vi "日志信息出发送队列 (子VI).vi"() -> (0 "错误输出":errorcluster)   [LabVIEW 2016, in "数据传输系统-05.lvlib"]
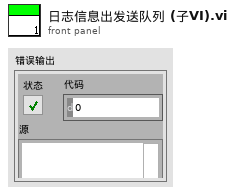
[diagram p1: front panel]
types:
  T1 = enum16{"空白测试", "跨度核查", "标样核查", "加标回收", "平行样", "集成干预"}
  T2 = cluster{"氨氮零点核查索引起始时间":string, "总磷零点核查索引起始时间":string, "总氮零点核查索引起始时间":string, "CODMn零点核查索引起始时间":string, "CODCr零点核查索引起始时间":string, "亚硝酸盐零点核查索引起始时间":string, "硫化物零点核查索引起始时间":string, "ORP零点核查索引起始时间":string, "氟化物零点核查索引起始时间":string}
  T3 = cluster{"数组[0]":string, "数组[1]":string, "数组[2]":string, "数组[3]":string, "数组[4]":string, "数组[5]":string, "数组[6]":string, "数组[7]":string, "数组[8]":string}
  T4 = cluster{"PH":string[][], "CODCr":string[][], "氨氮":string[][], "CODMn":string[][], "总氮":string[][], "总磷":string[][], "电导率":string[][], "水温":string[][], "DO":string[][], "浊度":string[][], "叶绿素":string[][], "藻密度":string[][], "铜":string[][], "盐度":string[][], "水位":string[][], "流速":string[][], "瞬时流量":string[][], "累积流量":string[][], "亚硝酸盐":string[][], "硫化物":string[][], "ORP":string[][], "铅":string[][], "镉":string[][], "锌":string[][], "镍":string[][], "锰":string[][], "汞":string[][], "气温":string[][], "气压":string[][], "风速":string[][], "风向":string[][], "盐度 2":string[][], "磷酸盐":string[][], "硝氮":string[][], "氟化物":string[][]}
  T5 = cluster{"氨氮跨度核查索引起始时间":string, "总磷跨度核查索引起始时间":string, "总氮跨度核查索引起始时间":string, "CODMn跨度核查索引起始时间":string, "CODCr跨度核查索引起始时间":string, "亚硝酸盐跨度核查索引起始时间":string, "硫化物跨度核查索引起始时间":string, "ORP跨度核查索引起始时间":string, "氟化物跨度核查索引起始时间":string}
  T6 = cluster{"氨氮标样核查索引起始时间":string, "总磷标样核查索引起始时间":string, "总氮标样核查索引起始时间":string, "CODMn标样核查索引起始时间":string, "CODCr标样核查索引起始时间":string, "DO标样核查索引起始时间":string, "PH标样核查索引起始时间":string, "比电导率标样核查索引起始时间":string, "水温标样核查索引起始时间":string, "浊度标样核查索引起始时间":string, "叶绿素a标样核查索引起始时间":string, "藻密度标样核查索引起始时间":string, "亚硝酸盐标样核查索引起始时间":string, "硫化物标样核查索引起始时间":string, "ORP标样核查索引起始时间":string, "氟化物标样核查索引起始时间":string}
  T7 = cluster{"数组[0]":string, "数组[1]":string, "数组[2]":string, "数组[3]":string, "数组[4]":string, "数组[5]":string, "数组[6]":string, "数组[7]":string, "数组[8]":string, "数组[9]":string, "数组[10]":string, "数组[11]":string, "数组[12]":string, "数组[13]":string, "数组[14]":string, "数组[15]":string}
  T8 = cluster{"氨氮加标回收索引起始时间":string, "总磷加标回收索引起始时间":string, "总氮加标回收索引起始时间":string, "CODMn加标回收索引起始时间":string, "CODCr加标回收索引起始时间":string, "氟化物加标回收索引起始时间":string}
  T9 = cluster{"[0]":string, "[1]":string, "[2]":string, "[3]":string, "[4]":string, "[5]":string}
  T10 = cluster{"氨氮平行样索引起始时间":string, "总磷平行样索引起始时间":string, "总氮平行样索引起始时间":string, "CODMn平行样索引起始时间":string, "CODCr平行样索引起始时间":string, "氟化物平行样索引起始时间":string}
  T11 = cluster{"氨氮集成干预索引起始时间":string, "总磷集成干预索引起始时间":string, "总氮集成干预索引起始时间":string, "CODMn集成干预索引起始时间":string, "CODCr集成干预索引起始时间":string, "DO集成干预索引起始时间":string, "PH集成干预索引起始时间":string, "比电导率集成干预索引起始时间":string, "水温集成干预索引起始时间":string, "浊度集成干预索引起始时间":string, "叶绿素a集成干预索引起始时间":string, "藻密度集成干预索引起始时间":string, "亚硝酸盐集成干预索引起始时间":string, "硫化物集成干预索引起始时间":string, "ORP集成干预索引起始时间":string, "氟化物集成干预索引起始时间":string}
  T12 = cluster{"[0]":string, "[1]":string, "[2]":string, "[3]":string, "[4]":string, "[5]":string, "[6]":string, "[7]":string, "[8]":string, "[9]":string, "[10]":string, "[11]":string, "[12]":string, "[13]":string, "[14]":string, "[15]":string}
  T13 = cluster{"氨氮仪器日志索引起始时间":string, "总磷仪器日志索引起始时间":string, "总氮仪器日志索引起始时间":string, "CODMn仪器日志索引起始时间":string, "CODCr仪器日志索引起始时间":string, "系统仪器日志索引起始时间":string, "氟化物仪器日志索引起始时间":string}
  T14 = cluster{"[0]":string, "[1]":string, "[2]":string, "[3]":string, "[4]":string, "[5]":string, "[6]":string}
  T15 = cluster{"氨氮报警信息索引起始时间":string, "总磷报警信息索引起始时间":string, "总氮报警信息索引起始时间":string, "CODMn报警信息索引起始时间":string, "CODCr报警信息索引起始时间":string, "DO报警信息索引起始时间":string, "PH报警信息索引起始时间":string, "比电导率报警信息索引起始时间":string, "水温报警信息索引起始时间":string, "浊度报警信息索引起始时间":string, "叶绿素报警信息索引起始时间":string, "系统报警信息索引起始时间":string, "氟化物报警信息索引起始时间":string}
  T16 = cluster{"[0]":string, "[1]":string, "[2]":string, "[3]":string, "[4]":string, "[5]":string, "[6]":string, "[7]":string, "[8]":string, "[9]":string, "[10]":string, "[11]":string, "[12]":string}
  T17 = cluster{"氨氮仪器参数索引起始时间":string, "总磷仪器参数索引起始时间":string, "总氮仪器参数索引起始时间":string, "CODMn仪器参数索引起始时间":string, "CODCr仪器参数索引起始时间":string, "DO仪器参数索引起始时间":string, "PH仪器参数索引起始时间":string, "比电导率仪器参数索引起始时间":string, "水温仪器参数索引起始时间":string, "浊度仪器参数索引起始时间":string, "叶绿素a仪器参数索引起始时间":string, "藻密度仪器参数索引起始时间":string, "ORP仪器参数索引起始时间":string, "氟化物仪器参数索引起始时间":string}
  T18 = cluster{"[0]":string, "[1]":string, "[2]":string, "[3]":string, "[4]":string, "[5]":string, "[6]":string, "[7]":string, "[8]":string, "[9]":string, "[10]":string, "[11]":string, "[12]":string, "[13]":string}
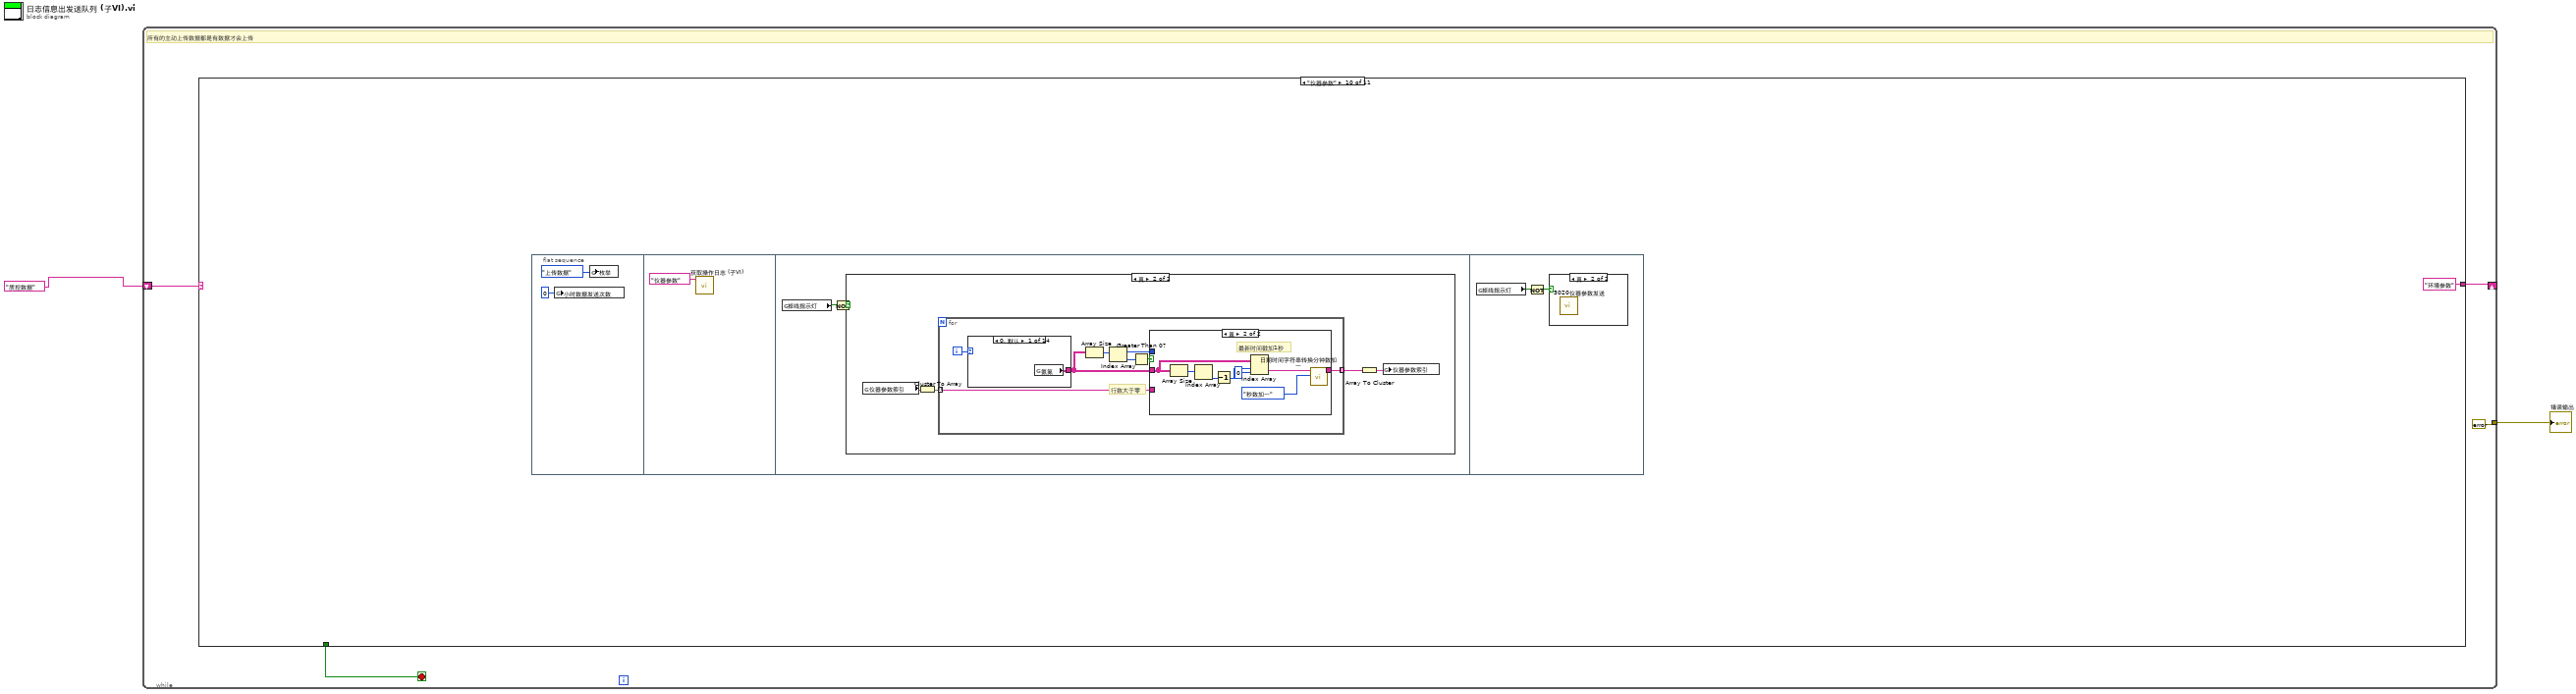
[diagram p0: block diagram]
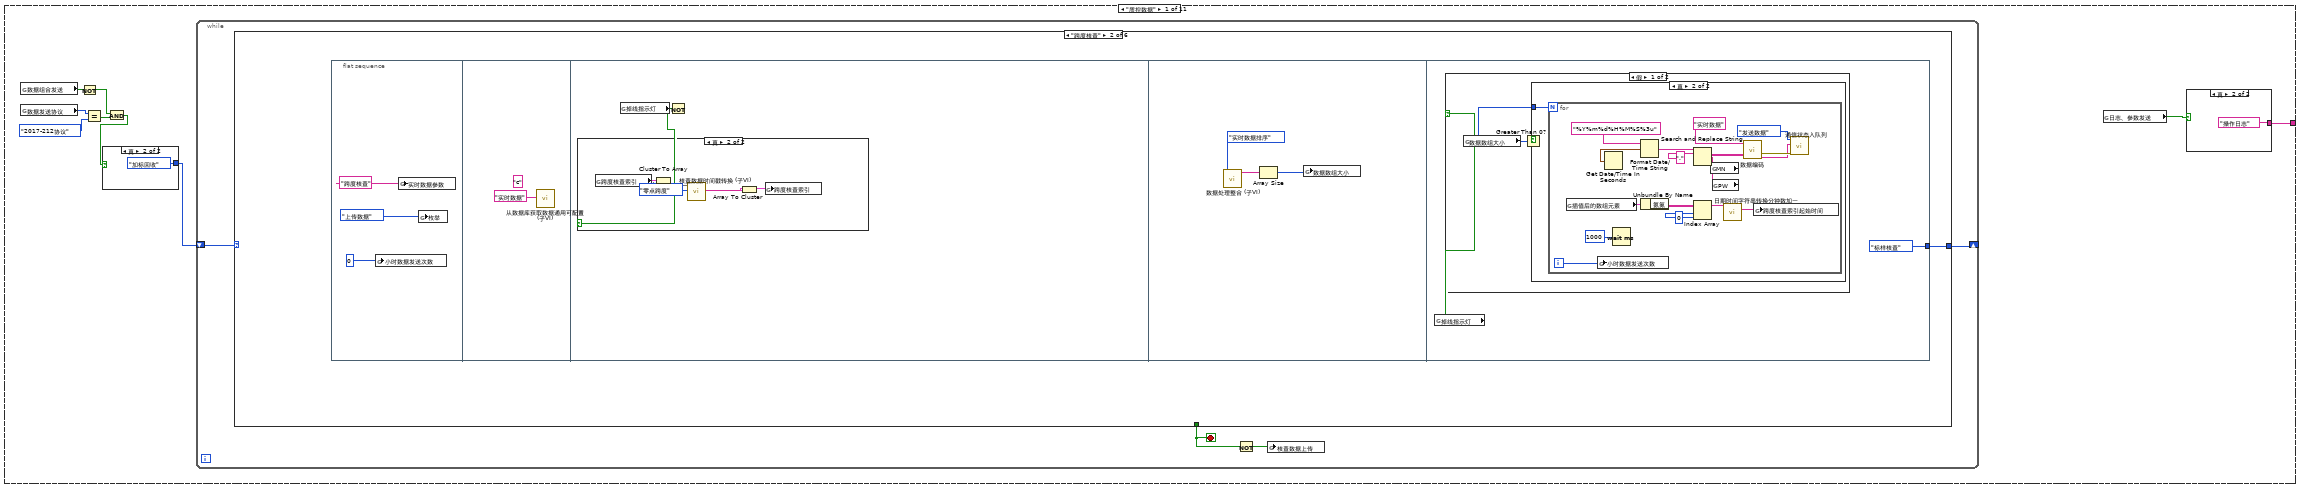
[diagram p2: hidden frame]
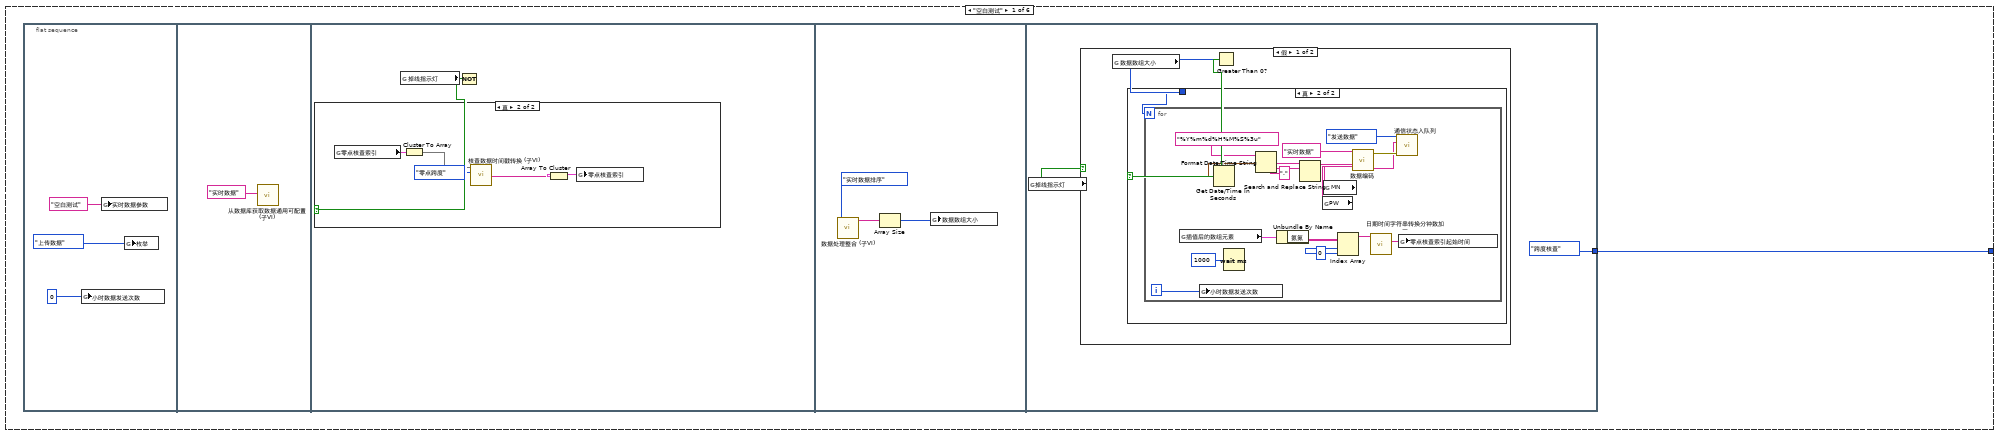
[diagram p3: hidden frame]
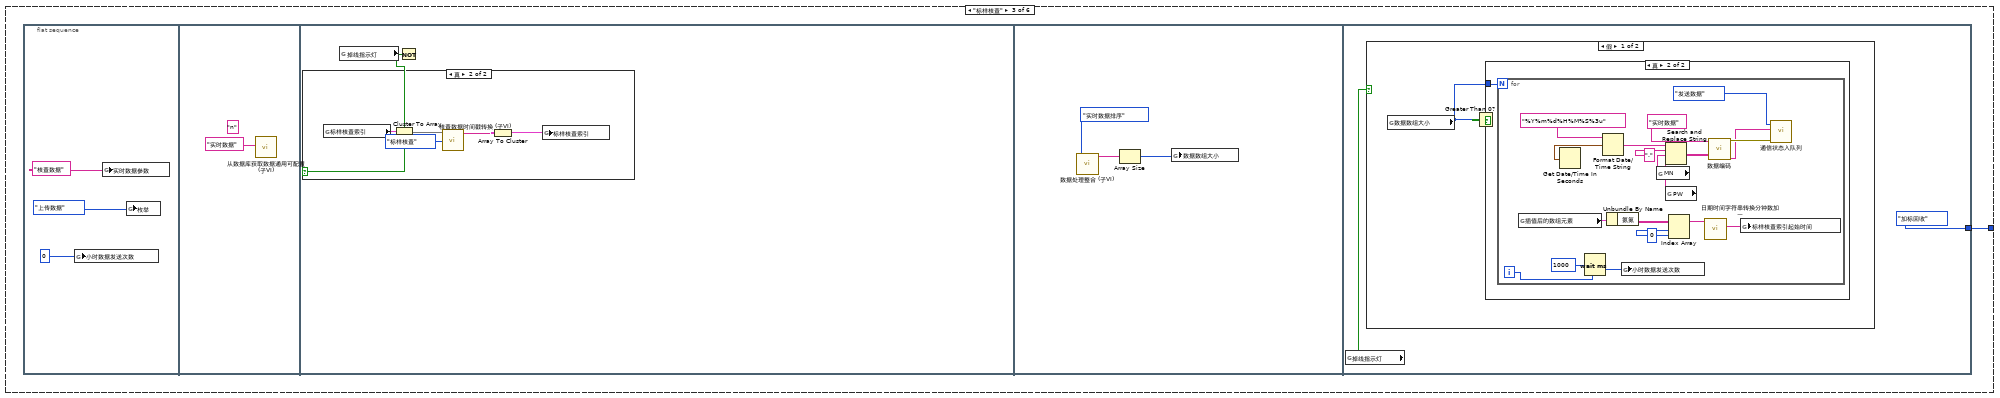
[diagram p10: hidden frame]
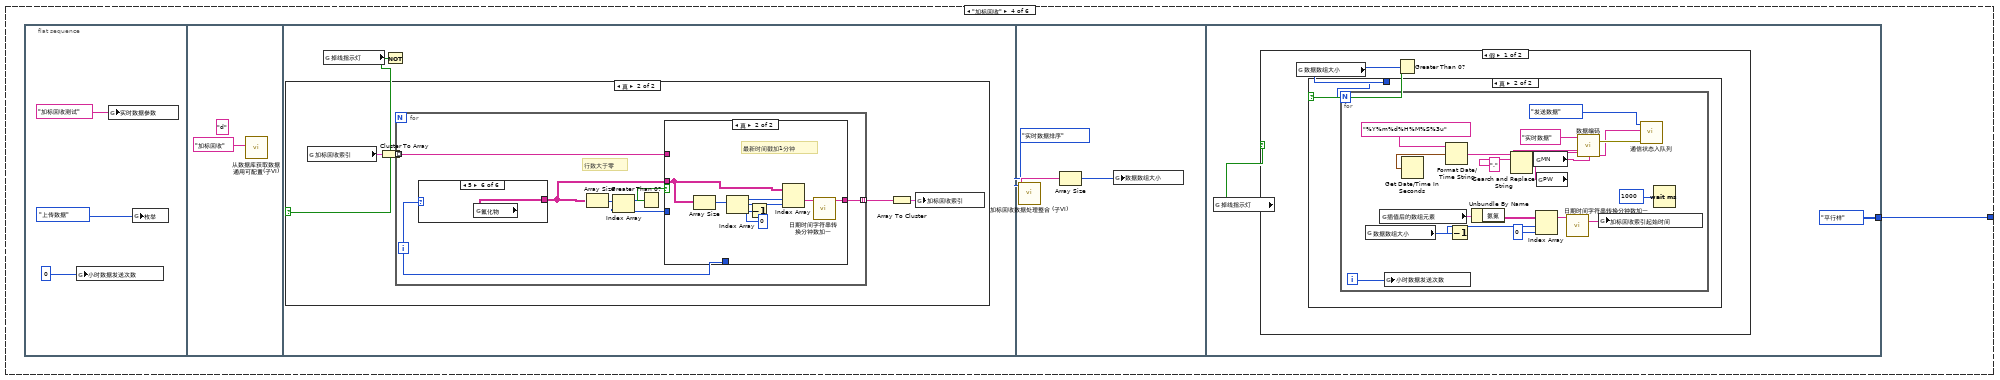
[diagram p14: hidden frame]
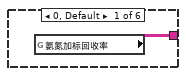
[diagram p16: hidden frame]
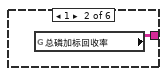
[diagram p17: hidden frame]
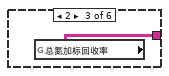
[diagram p18: hidden frame]
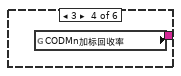
[diagram p19: hidden frame]
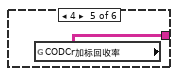
[diagram p20: hidden frame]
diagram:
  n1 = while "While循环" {
    shift-right: [w5] -> _
    shift-left: "质控数据" ("组合框") -> [w6]
    tunnel: [errorcluster {"status"=FALSE, "code"=0, "source"=""} ("错误输出")] -> w2
    stop <- w3 stop-if-true
    # "所有的主动上传数据都是有数据才会上传"
    n2 = case shown="\"仪器参数\"" w6 {
      tunnel: [w15 w315 "系统状态" ("组合框") w417 "测量周期" ("组合框") "超标留样" ("组合框") "报警信息" ("组合框") w559 w625 "环境参数" ("组合框") "环境参数" ("组合框")] -> w5
      tunnel: [_ _ _ _ _ _ _ _ _ _ TRUE] -> w3
      frame "质控数据" {
        n3 = global read "断电保存全局.vi" "数据组合发送"() -> (w10:bool)
        n4 = global read "断电保存全局.vi" "数据发送协议"() -> (w13:enum16{"2005-212协议", "2017-212协议"})
        n5 = Not(x=w10) -> (.not. x?=w9:bool)
        n6 = Equal?(x=w13, y=enum16{"2005-212协议", "2017-212协议"}."2017-212协议" ("数据发送协议")) -> (x = y?=w11:bool)
        n7 = And(x=w9, y=w11) -> (x .and. y?=w8:bool)
        n8 = case shown="真" w8 {
          tunnel: [T1."空白测试" T1."加标回收"] -> w7
          frame False {
          }
          frame True {
          }
        }
        n9 = while {
          shift-right: [w18] -> _
          shift-left: w7 -> [w19]
          stop <- w16 stop-if-true
          n10 = case shown="\"跨度核查\"" w19 {
            tunnel: [_ _ _ _ _ TRUE] -> w16
            tunnel: [w20 w58 w96 w134 w194 w247] -> w18
            frame "空白测试" {
              n11 = flat-sequence {
                tunnel: [T1."跨度核查"] -> w20
                frame #0 {
                  n12 = global write "全局 小时数据发送次数.vi" "小时数据发送次数"(0 ("小时数据发送次数")) -> ()
                  n13 = global write "全局 实时数据参数.vi" "实时数据参数"("空白测试") -> ()
                  n14 = global write "全局1.vi" "枚举"(enum16{"返回请求应答", "上传数据", "返回执行结果"}."上传数据" ("枚举")) -> ()
                }
                frame #1 {
                  n15 = call "从数据库获取数据通用可配置(子VI).vi"("table输入"="实时数据" ("新元素/子数组")) -> ()  [unwired: 9 in, 2 out]
                }
                frame #2 {
                  n16 = global read "全局 数据发送重叠.vi" "掉线指示灯"() -> (w26:bool)
                  n17 = Not(x=w26) -> (.not. x?=w25:bool)
                  n18 = case shown="真" w25 {
                    frame False {
                    }
                    frame True {
                      n19 = global read "全局 时间2.vi" "零点核查索引"() -> (w31:T2)
                      n20 = Cluster To Array(cluster=w31) -> (array=w29:string[])
                      n21 = call "核查数据时间戳转换 (子VI).vi"("枚举"=enum16{"零点跨度", "标样核查"}."零点跨度", "核查索引"=w29) -> ("数组"=w28:string[])  [unwired: 9 in]
                      n22 = Array To Cluster(array=w28) -> (cluster=w30:T3)
                      n23 = global write "全局 时间2.vi" "零点核查索引"(w30) -> ()
                    }
                  }
                }
                frame #3 {
                  n24 = call "数据处理整合 (子VI).vi"("枚举"=enum16{"实时数据排序", "小时数据排序"}."实时数据排序") -> ("已排序的数组"=w34:string[])  [unwired: 10 in]
                  n25 = Array Size(array=w34) -> (size(s)=w33:i32)
                  n26 = global write "全局 数据数组大小.vi" "数据数组大小"(w33) -> ()
                }
                frame #4 {
                  n27 = global read "全局 数据发送重叠.vi" "掉线指示灯"() -> (w36:bool)
                  n28 = case shown="假" w36 {
                    frame False {
                      n29 = global read "全局 数据数组大小.vi" "数据数组大小"() -> (w37:i32)
                      n30 = Greater Than 0?(x=w37) -> (x > 0?=w38:bool)
                      n31 = case shown="真" w38 {
                        tunnel: w37 -> [_ w39]
                        frame False {
                        }
                        frame True {
                          n32 = for {
                            N: w39 -> [_]
                            i -> [w42]
                            w52 = 0 ("禁用的索引 (列)")
                            n33 = global read "插值后的新数组.vi" "插值后的数组元素"() -> (w56:T4)
                            n34 = global write "全局 小时数据发送次数.vi" "小时数据发送次数"(w42) -> ()
                            n35 = Get Date/Time In Seconds() -> (seconds since 1Jan1904=w46:timestamp)
                            n36 = Wait (ms)(milliseconds to wait=u32 1000 ("等待时间（毫秒）")) -> ()  [unwired: 1 out]
                            n37 = Format Date/Time String(time format string (%c)="%Y%m%d%H%M%S%3u" ("时间格式字符串(%c)"), seconds (now)=w46) -> (date/time string=w45:string)  [unwired: 1 in]
                            n38 = Unbundle By Name(w56) -> ("氨氮"=w55:string[][])
                            n39 = Search and Replace String(input string=w45, search string="." ("搜索字符串")) -> (result string=w43:string)  [unwired: 6 in, 3 out]
                            n40 = global read "断电保存全局.vi" "PW"() -> (w50:string)
                            n41 = global read "断电保存全局.vi" "MN"() -> (w51:string)
                            n42 = Index Array(array=w55, index (row)=w52, index (col)=w52) -> (element=w54:string)
                            n43 = call "数据编码.vi"("table输入"="实时数据" ("新元素/子数组"), "QN"=w43, "MN"=w51, "PW"=w50) -> ("错误常量"=w49:errorcluster, "通讯包字符串"=w40:string)  [unwired: 10 in]
                            n44 = call "日期时间字符串转换分钟数加一.vi"("data[0]"=w54) -> ("日期/时间字符串"=w53:string)  [unwired: 10 in]
                            n45 = call "通信状态入队列.vi"("错误输入（无错误）"=w49, "发送报文"=w40, "枚举"=enum16{"打开连接", "发送数据", "读取数据", "数据处理", "关闭连接"}."发送数据") -> ()  [unwired: 8 in, 1 out]
                            n46 = global write "全局 时间2.vi" "零点核查索引起始时间"(w53) -> ()
                          }
                        }
                      }
                    }
                    frame True {
                    }
                  }
                }
              }
            }
            frame "跨度核查" {
              n47 = flat-sequence {
                tunnel: [T1."标样核查"] -> w58
                frame #0 {
                  n48 = global write "全局 小时数据发送次数.vi" "小时数据发送次数"(0 ("小时数据发送次数")) -> ()
                  n49 = global write "全局 实时数据参数.vi" "实时数据参数"("跨度核查") -> ()
                  n50 = global write "全局1.vi" "枚举"(enum16{"返回请求应答", "上传数据", "返回执行结果"}."上传数据" ("枚举")) -> ()
                }
                frame #1 {
                  (unwired) "c" ("列队名（唯一）")
                  n51 = call "从数据库获取数据通用可配置(子VI).vi"("table输入"="实时数据" ("新元素/子数组")) -> ()  [unwired: 9 in, 2 out]
                }
                frame #2 {
                  n52 = global read "全局 数据发送重叠.vi" "掉线指示灯"() -> (w64:bool)
                  n53 = Not(x=w64) -> (.not. x?=w63:bool)
                  n54 = case shown="真" w63 {
                    frame False {
                    }
                    frame True {
                      n55 = global read "全局 时间2.vi" "跨度核查索引"() -> (w69:T5)
                      n56 = Cluster To Array(cluster=w69) -> (array=w67:string[])
                      n57 = call "核查数据时间戳转换 (子VI).vi"("枚举"=enum16{"零点跨度", "标样核查"}."零点跨度", "核查索引"=w67) -> ("数组"=w66:string[])  [unwired: 9 in]
                      n58 = Array To Cluster(array=w66) -> (cluster=w68:T3)
                      n59 = global write "全局 时间2.vi" "跨度核查索引"(w68) -> ()
                    }
                  }
                }
                frame #3 {
                  n60 = call "数据处理整合 (子VI).vi"("枚举"=enum16{"实时数据排序", "小时数据排序"}."实时数据排序") -> ("已排序的数组"=w72:string[])  [unwired: 10 in]
                  n61 = Array Size(array=w72) -> (size(s)=w71:i32)
                  n62 = global write "全局 数据数组大小.vi" "数据数组大小"(w71) -> ()
                }
                frame #4 {
                  n63 = global read "全局 数据发送重叠.vi" "掉线指示灯"() -> (w74:bool)
                  n64 = case shown="假" w74 {
                    frame False {
                      n65 = global read "全局 数据数组大小.vi" "数据数组大小"() -> (w75:i32)
                      n66 = Greater Than 0?(x=w75) -> (x > 0?=w76:bool)
                      n67 = case shown="真" w76 {
                        tunnel: w75 -> [_ w77]
                        frame False {
                        }
                        frame True {
                          n68 = for {
                            N: w77 -> [_]
                            i -> [w80]
                            w90 = 0 ("禁用的索引 (列)")
                            n69 = global read "插值后的新数组.vi" "插值后的数组元素"() -> (w94:T4)
                            n70 = global write "全局 小时数据发送次数.vi" "小时数据发送次数"(w80) -> ()
                            n71 = Get Date/Time In Seconds() -> (seconds since 1Jan1904=w84:timestamp)
                            n72 = Wait (ms)(milliseconds to wait=u32 1000 ("等待时间（毫秒）")) -> ()  [unwired: 1 out]
                            n73 = Format Date/Time String(time format string (%c)="%Y%m%d%H%M%S%3u" ("时间格式字符串(%c)"), seconds (now)=w84) -> (date/time string=w83:string)  [unwired: 1 in]
                            n74 = Unbundle By Name(w94) -> ("氨氮"=w93:string[][])
                            n75 = Index Array(array=w93, index (row)=w90, index (col)=w90) -> (element=w92:string)
                            n76 = Search and Replace String(input string=w83, search string="." ("搜索字符串")) -> (result string=w81:string)  [unwired: 6 in, 3 out]
                            n77 = global read "断电保存全局.vi" "MN"() -> (w89:string)
                            n78 = global read "断电保存全局.vi" "PW"() -> (w88:string)
                            n79 = call "日期时间字符串转换分钟数加一.vi"("data[0]"=w92) -> ("日期/时间字符串"=w91:string)  [unwired: 10 in]
                            n80 = call "数据编码.vi"("table输入"="实时数据" ("新元素/子数组"), "QN"=w81, "MN"=w89, "PW"=w88) -> ("错误常量"=w87:errorcluster, "通讯包字符串"=w78:string)  [unwired: 10 in]
                            n81 = global write "全局 时间2.vi" "跨度核查索引起始时间"(w91) -> ()
                            n82 = call "通信状态入队列.vi"("错误输入（无错误）"=w87, "发送报文"=w78, "枚举"=enum16{"打开连接", "发送数据", "读取数据", "数据处理", "关闭连接"}."发送数据") -> ()  [unwired: 8 in, 1 out]
                          }
                        }
                      }
                    }
                    frame True {
                    }
                  }
                }
              }
            }
            frame "标样核查" {
              n83 = flat-sequence {
                tunnel: [T1."加标回收"] -> w96
                frame #0 {
                  n84 = global write "全局 小时数据发送次数.vi" "小时数据发送次数"(0 ("小时数据发送次数")) -> ()
                  n85 = global write "全局 实时数据参数.vi" "实时数据参数"("核查数据") -> ()
                  n86 = global write "全局1.vi" "枚举"(enum16{"返回请求应答", "上传数据", "返回执行结果"}."上传数据" ("枚举")) -> ()
                }
                frame #1 {
                  (unwired) "n" ("列队名（唯一）")
                  n87 = call "从数据库获取数据通用可配置(子VI).vi"("table输入"="实时数据" ("新元素/子数组")) -> ()  [unwired: 9 in, 2 out]
                }
                frame #2 {
                  n88 = global read "全局 数据发送重叠.vi" "掉线指示灯"() -> (w102:bool)
                  n89 = Not(x=w102) -> (.not. x?=w101:bool)
                  n90 = case shown="真" w101 {
                    frame False {
                    }
                    frame True {
                      n91 = global read "全局 时间2.vi" "标样核查索引"() -> (w107:T6)
                      n92 = Cluster To Array(cluster=w107) -> (array=w105:string[])
                      n93 = call "核查数据时间戳转换 (子VI).vi"("枚举"=enum16{"零点跨度", "标样核查"}."标样核查", "核查索引"=w105) -> ("数组"=w104:string[])  [unwired: 9 in]
                      n94 = Array To Cluster(array=w104) -> (cluster=w106:T7)
                      n95 = global write "全局 时间2.vi" "标样核查索引"(w106) -> ()
                    }
                  }
                }
                frame #3 {
                  n96 = call "数据处理整合 (子VI).vi"("枚举"=enum16{"实时数据排序", "小时数据排序"}."实时数据排序") -> ("已排序的数组"=w110:string[])  [unwired: 10 in]
                  n97 = Array Size(array=w110) -> (size(s)=w109:i32)
                  n98 = global write "全局 数据数组大小.vi" "数据数组大小"(w109) -> ()
                }
                frame #4 {
                  n99 = global read "全局 数据发送重叠.vi" "掉线指示灯"() -> (w112:bool)
                  n100 = case shown="假" w112 {
                    frame False {
                      n101 = global read "全局 数据数组大小.vi" "数据数组大小"() -> (w113:i32)
                      n102 = Greater Than 0?(x=w113) -> (x > 0?=w114:bool)
                      n103 = case shown="真" w114 {
                        tunnel: w113 -> [_ w115]
                        frame False {
                        }
                        frame True {
                          n104 = for {
                            N: w115 -> [_]
                            i -> [w118]
                            w128 = 0 ("禁用的索引 (列)")
                            n105 = global read "插值后的新数组.vi" "插值后的数组元素"() -> (w132:T4)
                            n106 = Get Date/Time In Seconds() -> (seconds since 1Jan1904=w122:timestamp)
                            n107 = Wait (ms)(milliseconds to wait=u32 1000 ("等待时间（毫秒）")) -> ()  [unwired: 1 out]
                            n108 = Format Date/Time String(time format string (%c)="%Y%m%d%H%M%S%3u" ("时间格式字符串(%c)"), seconds (now)=w122) -> (date/time string=w121:string)  [unwired: 1 in]
                            n109 = Unbundle By Name(w132) -> ("氨氮"=w131:string[][])
                            n110 = global write "全局 小时数据发送次数.vi" "小时数据发送次数"(w118) -> ()
                            n111 = global read "断电保存全局.vi" "MN"() -> (w127:string)
                            n112 = Search and Replace String(input string=w121, search string="." ("搜索字符串")) -> (result string=w119:string)  [unwired: 6 in, 3 out]
                            n113 = global read "断电保存全局.vi" "PW"() -> (w126:string)
                            n114 = Index Array(array=w131, index (row)=w128, index (col)=w128) -> (element=w130:string)
                            n115 = call "日期时间字符串转换分钟数加一.vi"("data[0]"=w130) -> ("日期/时间字符串"=w129:string)  [unwired: 10 in]
                            n116 = call "数据编码.vi"("table输入"="实时数据" ("新元素/子数组"), "QN"=w119, "MN"=w127, "PW"=w126) -> ("错误常量"=w125:errorcluster, "通讯包字符串"=w116:string)  [unwired: 10 in]
                            n117 = global write "全局 时间2.vi" "标样核查索引起始时间"(w129) -> ()
                            n118 = call "通信状态入队列.vi"("错误输入（无错误）"=w125, "发送报文"=w116, "枚举"=enum16{"打开连接", "发送数据", "读取数据", "数据处理", "关闭连接"}."发送数据") -> ()  [unwired: 8 in, 1 out]
                          }
                        }
                      }
                    }
                    frame True {
                    }
                  }
                }
              }
            }
            frame "加标回收" {
              n119 = flat-sequence {
                tunnel: [T1."平行样"] -> w134
                frame #0 {
                  n120 = global write "全局 小时数据发送次数.vi" "小时数据发送次数"(0 ("小时数据发送次数")) -> ()
                  n121 = global write "全局 实时数据参数.vi" "实时数据参数"("加标回收测试") -> ()
                  n122 = global write "全局1.vi" "枚举"(enum16{"返回请求应答", "上传数据", "返回执行结果"}."上传数据" ("枚举")) -> ()
                }
                frame #1 {
                  (unwired) "d" ("列队名（唯一）")
                  n123 = call "从数据库获取数据通用可配置(子VI).vi"("table输入"="加标回收" ("新元素/子数组")) -> ()  [unwired: 9 in, 2 out]
                }
                frame #2 {
                  n124 = global read "全局 数据发送重叠.vi" "掉线指示灯"() -> (w140:bool)
                  n125 = Not(x=w140) -> (.not. x?=w139:bool)
                  n126 = case shown="真" w139 {
                    frame False {
                    }
                    frame True {
                      n127 = global read "全局 时间2.vi" "加标回收索引"() -> (w144:T8)
                      n128 = Cluster To Array(cluster=w144) -> (array=w143:string[])
                      n129 = for {
                        tunnel: [w146] -> w141 mode=indexing
                        tunnel: w143 -> [w145] mode=indexing
                        i -> [w147]
                        # "行数大于零"
                        n130 = case shown="5" w147 {
                          tunnel: [w152 w153 w154 w155 w156 w157] -> w148
                          frame 0, Default {
                            n131 = global read "全局 所有参数.vi" "氨氮加标回收率"() -> (w152:string[][])
                          }
                          frame 1 {
                            n132 = global read "全局 所有参数.vi" "总磷加标回收率"() -> (w153:string[][])
                          }
                          frame 2 {
                            n133 = global read "全局 所有参数.vi" "总氮加标回收率"() -> (w154:string[][])
                          }
                          frame 3 {
                            n134 = global read "全局 所有参数.vi" "CODMn加标回收率"() -> (w155:string[][])
                          }
                          frame 4 {
                            n135 = global read "全局 所有参数.vi" "CODCr加标回收率"() -> (w156:string[][])
                          }
                          frame 5 {
                            n136 = global read "全局 所有参数.vi" "氟化物"() -> (w157:string[][])
                          }
                        }
                        n137 = Array Size(array=w148) -> (size(s)=w150:i32[])
                        n138 = Index Array(array=w150) -> (element=w149:i32)  [unwired: 1 in]
                        n139 = Greater Than 0?(x=w149) -> (x > 0?=w151:bool)
                        n140 = case shown="真" w151 {
                          tunnel: w147 -> [_ _]
                          tunnel: w149 -> [_ _]
                          tunnel: w148 -> [_ w162]
                          tunnel: [w158 w159] -> w146
                          tunnel: w145 -> [w158 _]
                          frame False {
                          }
                          frame True {
                            # "最新时间戳加1分钟"
                            n141 = Array Size(array=w162) -> (size(s)=w164:i32[])
                            n142 = Index Array(array=w164) -> (element=w163:i32)  [unwired: 1 in]
                            n143 = Decrement(x=w163) -> (x-1=w161:i32)
                            n144 = Index Array(array=w162, index (row)=w161, index (col)=0 ("禁用的索引 (列)")) -> (element=w165:string)
                            n145 = call "日期时间字符串转换分钟数加一.vi"("data[0]"=w165) -> ("日期/时间字符串"=w159:string)  [unwired: 10 in]
                          }
                        }
                      }
                      n146 = Array To Cluster(array=w141) -> (cluster=w142:T9)
                      n147 = global write "全局 时间2.vi" "加标回收索引"(w142) -> ()
                    }
                  }
                }
                frame #3 {
                  n148 = call "加标回收数据处理整合 (子VI).vi"("枚举"=enum16{"实时数据排序", "小时数据排序"}."实时数据排序") -> ("已排序的数组"=w167:string[])  [unwired: 10 in]
                  n149 = Array Size(array=w167) -> (size(s)=w168:i32)
                  n150 = global write "全局 数据数组大小.vi" "数据数组大小"(w168) -> ()
                }
                frame #4 {
                  n151 = global read "全局 数据发送重叠.vi" "掉线指示灯"() -> (w170:bool)
                  n152 = case shown="假" w170 {
                    frame False {
                      n153 = global read "全局 数据数组大小.vi" "数据数组大小"() -> (w171:i32)
                      n154 = Greater Than 0?(x=w171) -> (x > 0?=w172:bool)
                      n155 = case shown="真" w172 {
                        tunnel: w171 -> [_ w173]
                        frame False {
                        }
                        frame True {
                          n156 = for {
                            N: w173 -> [_]
                            i -> [w176]
                            n157 = global read "全局 数据数组大小.vi" "数据数组大小"() -> (w189:i32)
                            n158 = global read "插值后的新数组.vi" "插值后的数组元素"() -> (w192:T4)
                            n159 = global write "全局 小时数据发送次数.vi" "小时数据发送次数"(w176) -> ()
                            n160 = Get Date/Time In Seconds() -> (seconds since 1Jan1904=w180:timestamp)
                            n161 = Format Date/Time String(time format string (%c)="%Y%m%d%H%M%S%3u" ("时间格式字符串(%c)"), seconds (now)=w180) -> (date/time string=w179:string)  [unwired: 1 in]
                            n162 = Decrement(x=w189) -> (x-1=w188:i32)
                            n163 = Unbundle By Name(w192) -> ("氨氮"=w191:string[][])
                            n164 = Search and Replace String(input string=w179, search string="." ("搜索字符串")) -> (result string=w177:string)  [unwired: 6 in, 3 out]
                            n165 = global read "断电保存全局.vi" "MN"() -> (w185:string)
                            n166 = Index Array(array=w191, index (row)=w188, index (col)=0 ("禁用的索引 (列)")) -> (element=w187:string)
                            n167 = global read "断电保存全局.vi" "PW"() -> (w184:string)
                            n168 = call "日期时间字符串转换分钟数加一.vi"("data[0]"=w187) -> ("日期/时间字符串"=w186:string)  [unwired: 10 in]
                            n169 = call "数据编码.vi"("table输入"="实时数据" ("新元素/子数组"), "QN"=w177, "MN"=w185, "PW"=w184) -> ("错误常量"=w183:errorcluster, "通讯包字符串"=w174:string)  [unwired: 10 in]
                            n170 = global write "全局 时间2.vi" "加标回收索引起始时间"(w186) -> ()
                            n171 = call "通信状态入队列.vi"("错误输入（无错误）"=w183, "发送报文"=w174, "枚举"=enum16{"打开连接", "发送数据", "读取数据", "数据处理", "关闭连接"}."发送数据") -> ()  [unwired: 8 in, 1 out]
                            n172 = Wait (ms)(milliseconds to wait=u32 1000 ("等待时间（毫秒）")) -> ()  [unwired: 1 out]
                          }
                        }
                      }
                    }
                    frame True {
                    }
                  }
                }
              }
            }
            frame "平行样" {
              n173 = flat-sequence {
                tunnel: [T1."集成干预"] -> w194
                frame #0 {
                  n174 = global write "全局 小时数据发送次数.vi" "小时数据发送次数"(0 ("小时数据发送次数")) -> ()
                  n175 = global write "全局 实时数据参数.vi" "实时数据参数"("平行样测试") -> ()
                  n176 = global write "全局1.vi" "枚举"(enum16{"返回请求应答", "上传数据", "返回执行结果"}."上传数据" ("枚举")) -> ()
                }
                frame #1 {
                  (unwired) "e" ("列队名（唯一）")
                  n177 = call "从数据库获取数据通用可配置(子VI).vi"("table输入"="平行样测试" ("新元素/子数组")) -> ()  [unwired: 9 in, 2 out]
                }
                frame #2 {
                  n178 = global read "全局 数据发送重叠.vi" "掉线指示灯"() -> (w200:bool)
                  n179 = Not(x=w200) -> (.not. x?=w199:bool)
                  n180 = case shown="真" w199 {
                    frame False {
                    }
                    frame True {
                      n181 = global read "全局 时间2.vi" "平行样索引"() -> (w204:T10)
                      n182 = Cluster To Array(cluster=w204) -> (array=w203:string[])
                      n183 = for {
                        tunnel: [w206] -> w201 mode=indexing
                        tunnel: w203 -> [w205] mode=indexing
                        i -> [w207]
                        # "行数大于零"
                        n184 = case shown="5" w207 {
                          tunnel: [w212 w213 w214 w215 w216 w217] -> w208
                          frame 0, Default {
                            n185 = global read "全局 所有参数.vi" "氨氮"() -> (w212:string[][])
                          }
                          frame 1 {
                            n186 = global read "全局 所有参数.vi" "总磷"() -> (w213:string[][])
                          }
                          frame 2 {
                            n187 = global read "全局 所有参数.vi" "总氮"() -> (w214:string[][])
                          }
                          frame 3 {
                            n188 = global read "全局 所有参数.vi" "CODMn"() -> (w215:string[][])
                          }
                          frame 4 {
                            n189 = global read "全局 所有参数.vi" "CODCr"() -> (w216:string[][])
                          }
                          frame 5 {
                            n190 = global read "全局 所有参数.vi" "氟化物"() -> (w217:string[][])
                          }
                        }
                        n191 = Array Size(array=w208) -> (size(s)=w210:i32[])
                        n192 = Index Array(array=w210) -> (element=w209:i32)  [unwired: 1 in]
                        n193 = Greater Than 0?(x=w209) -> (x > 0?=w211:bool)
                        n194 = case shown="真" w211 {
                          tunnel: w207 -> [_ _]
                          tunnel: w209 -> [_ _]
                          tunnel: w208 -> [_ w222]
                          tunnel: [w218 w219] -> w206
                          tunnel: w205 -> [w218 _]
                          frame False {
                          }
                          frame True {
                            # "最新时间戳加1分钟"
                            n195 = Array Size(array=w222) -> (size(s)=w224:i32[])
                            n196 = Index Array(array=w224) -> (element=w223:i32)  [unwired: 1 in]
                            n197 = Decrement(x=w223) -> (x-1=w221:i32)
                            n198 = Index Array(array=w222, index (row)=w221, index (col)=0 ("禁用的索引 (列)")) -> (element=w225:string)
                            n199 = call "日期时间字符串转换分钟数加一.vi"("data[0]"=w225) -> ("日期/时间字符串"=w219:string)  [unwired: 10 in]
                          }
                        }
                      }
                      n200 = Array To Cluster(array=w201) -> (cluster=w202:T9)
                      n201 = global write "全局 时间2.vi" "平行样索引"(w202) -> ()
                    }
                  }
                }
                frame #3 {
                  n202 = call "数据处理整合 (子VI).vi"("枚举"=enum16{"实时数据排序", "小时数据排序"}."实时数据排序") -> ("已排序的数组"=w228:string[])  [unwired: 10 in]
                  n203 = Array Size(array=w228) -> (size(s)=w227:i32)
                  n204 = global write "全局 数据数组大小.vi" "数据数组大小"(w227) -> ()
                }
                frame #4 {
                  n205 = global read "全局 数据发送重叠.vi" "掉线指示灯"() -> (w229:bool)
                  n206 = case shown="假" w229 {
                    frame False {
                      n207 = global read "全局 数据数组大小.vi" "数据数组大小"() -> (w231:i32)
                      n208 = Greater Than 0?(x=w231) -> (x > 0?=w232:bool)
                      n209 = case shown="真" w232 {
                        tunnel: w231 -> [_ w233]
                        frame False {
                        }
                        frame True {
                          n210 = for {
                            N: w233 -> [_]
                            i -> [w236]
                            n211 = global write "全局 小时数据发送次数.vi" "小时数据发送次数"(w236) -> ()
                            n212 = Get Date/Time In Seconds() -> (seconds since 1Jan1904=w240:timestamp)
                            n213 = Format Date/Time String(time format string (%c)="%Y%m%d%H%M%S%3u" ("时间格式字符串(%c)"), seconds (now)=w240) -> (date/time string=w239:string)  [unwired: 1 in]
                            n214 = Search and Replace String(input string=w239, search string="." ("搜索字符串")) -> (result string=w237:string)  [unwired: 6 in, 3 out]
                            n215 = global read "断电保存全局.vi" "MN"() -> (w245:string)
                            n216 = global read "断电保存全局.vi" "PW"() -> (w244:string)
                            n217 = call "数据编码.vi"("table输入"="实时数据" ("新元素/子数组"), "QN"=w237, "MN"=w245, "PW"=w244) -> ("错误常量"=w243:errorcluster, "通讯包字符串"=w234:string)  [unwired: 10 in]
                            n218 = call "通信状态入队列.vi"("错误输入（无错误）"=w243, "发送报文"=w234, "枚举"=enum16{"打开连接", "发送数据", "读取数据", "数据处理", "关闭连接"}."发送数据") -> ()  [unwired: 8 in, 1 out]
                            n219 = Wait (ms)(milliseconds to wait=u32 1000 ("等待时间（毫秒）")) -> ()  [unwired: 1 out]
                          }
                        }
                      }
                    }
                    frame True {
                    }
                  }
                }
              }
            }
            frame "集成干预" {
              n220 = flat-sequence {
                tunnel: [T1."集成干预"] -> w247
                frame #0 {
                  n221 = global write "全局 小时数据发送次数.vi" "小时数据发送次数"(0 ("小时数据发送次数")) -> ()
                  n222 = global write "全局 实时数据参数.vi" "实时数据参数"("集成干预测试") -> ()
                  n223 = global write "全局1.vi" "枚举"(enum16{"返回请求应答", "上传数据", "返回执行结果"}."上传数据" ("枚举")) -> ()
                }
                frame #1 {
                  (unwired) "f" ("列队名（唯一）")
                  n224 = call "从数据库获取数据通用可配置(子VI).vi"("table输入"="集成干预测试" ("新元素/子数组")) -> ()  [unwired: 9 in, 2 out]
                }
                frame #2 {
                  n225 = global read "全局 数据发送重叠.vi" "掉线指示灯"() -> (w254:bool)
                  n226 = Not(x=w254) -> (.not. x?=w253:bool)
                  n227 = case shown="真" w253 {
                    frame False {
                    }
                    frame True {
                      n228 = global read "全局 时间2.vi" "集成干预索引"() -> (w258:T11)
                      n229 = Cluster To Array(cluster=w258) -> (array=w257:string[])
                      n230 = for {
                        tunnel: [w260] -> w255 mode=indexing
                        tunnel: w257 -> [w259] mode=indexing
                        i -> [w261]
                        # "行数大于零"
                        n231 = case shown="15" w261 {
                          tunnel: [w266 w267 w268 w269 w270 w271 w272 w273 w274 w275 w276 w277 w278 w279 w280 w281] -> w262
                          frame 0, Default {
                            n232 = global read "全局 所有参数.vi" "氨氮"() -> (w266:string[][])
                          }
                          frame 1 {
                            n233 = global read "全局 所有参数.vi" "总磷"() -> (w267:string[][])
                          }
                          frame 2 {
                            n234 = global read "全局 所有参数.vi" "总氮"() -> (w268:string[][])
                          }
                          frame 3 {
                            n235 = global read "全局 所有参数.vi" "CODMn"() -> (w269:string[][])
                          }
                          frame 4 {
                            n236 = global read "全局 所有参数.vi" "CODCr"() -> (w270:string[][])
                          }
                          frame 5 {
                            n237 = global read "全局 所有参数.vi" "DO"() -> (w271:string[][])
                          }
                          frame 6 {
                            n238 = global read "全局 所有参数.vi" "PH"() -> (w272:string[][])
                          }
                          frame 7 {
                            n239 = global read "全局 所有参数.vi" "电导率"() -> (w273:string[][])
                          }
                          frame 8 {
                            n240 = global read "全局 所有参数.vi" "水温"() -> (w274:string[][])
                          }
                          frame 9 {
                            n241 = global read "全局 所有参数.vi" "浊度"() -> (w275:string[][])
                          }
                          frame 10 {
                            n242 = global read "全局 所有参数.vi" "叶绿素"() -> (w276:string[][])
                          }
                          frame 11 {
                            n243 = global read "全局 所有参数.vi" "藻密度"() -> (w277:string[][])
                          }
                          frame 12 {
                            n244 = global read "全局 所有参数.vi" "亚硝酸盐"() -> (w278:string[][])
                          }
                          frame 13 {
                            n245 = global read "全局 所有参数.vi" "硫化物"() -> (w279:string[][])
                          }
                          frame 14 {
                            n246 = global read "全局 所有参数.vi" "ORP"() -> (w280:string[][])
                          }
                          frame 15 {
                            n247 = global read "全局 所有参数.vi" "氟化物"() -> (w281:string[][])
                          }
                        }
                        n248 = Array Size(array=w262) -> (size(s)=w264:i32[])
                        n249 = Index Array(array=w264) -> (element=w263:i32)  [unwired: 1 in]
                        n250 = Greater Than 0?(x=w263) -> (x > 0?=w265:bool)
                        n251 = case shown="真" w265 {
                          tunnel: w261 -> [_ _]
                          tunnel: w263 -> [_ _]
                          tunnel: w262 -> [_ w284]
                          tunnel: [w282 w283] -> w260
                          tunnel: w259 -> [w282 _]
                          frame False {
                          }
                          frame True {
                            # "最新时间戳加1分钟"
                            n252 = Array Size(array=w284) -> (size(s)=w288:i32[])
                            n253 = Index Array(array=w288) -> (element=w287:i32)  [unwired: 1 in]
                            n254 = Decrement(x=w287) -> (x-1=w286:i32)
                            n255 = Index Array(array=w284, index (row)=w286, index (col)=0 ("禁用的索引 (列)")) -> (element=w289:string)
                            n256 = call "日期时间字符串转换分钟数加一.vi"("data[0]"=w289) -> ("日期/时间字符串"=w283:string)  [unwired: 10 in]
                          }
                        }
                      }
                      n257 = Array To Cluster(array=w255) -> (cluster=w256:T12)
                      n258 = global write "全局 时间2.vi" "集成干预索引"(w256) -> ()
                    }
                  }
                }
                frame #3 {
                  n259 = call "数据处理整合 (子VI).vi"("枚举"=enum16{"实时数据排序", "小时数据排序"}."实时数据排序") -> ("已排序的数组"=w292:string[])  [unwired: 10 in]
                  n260 = Array Size(array=w292) -> (size(s)=w291:i32)
                  n261 = global write "全局 数据数组大小.vi" "数据数组大小"(w291) -> ()
                }
                frame #4 {
                  n262 = global read "全局 数据发送重叠.vi" "掉线指示灯"() -> (w294:bool)
                  n263 = case shown="假" w294 {
                    frame False {
                      n264 = global read "全局 数据数组大小.vi" "数据数组大小"() -> (w295:i32)
                      n265 = Greater Than 0?(x=w295) -> (x > 0?=w296:bool)
                      n266 = case shown="真" w296 {
                        tunnel: w295 -> [_ w297]
                        frame False {
                        }
                        frame True {
                          n267 = for {
                            N: w297 -> [_]
                            i -> [w300]
                            n268 = Get Date/Time In Seconds() -> (seconds since 1Jan1904=w304:timestamp)
                            n269 = Format Date/Time String(time format string (%c)="%Y%m%d%H%M%S%3u" ("时间格式字符串(%c)"), seconds (now)=w304) -> (date/time string=w303:string)  [unwired: 1 in]
                            n270 = global write "全局 小时数据发送次数.vi" "小时数据发送次数"(w300) -> ()
                            n271 = global read "断电保存全局.vi" "MN"() -> (w308:string)
                            n272 = global read "断电保存全局.vi" "PW"() -> (w307:string)
                            n273 = Search and Replace String(input string=w303, search string="." ("搜索字符串")) -> (result string=w301:string)  [unwired: 6 in, 3 out]
                            n274 = call "数据编码.vi"("table输入"="实时数据" ("新元素/子数组"), "QN"=w301, "MN"=w308, "PW"=w307) -> ("错误常量"=w309:errorcluster, "通讯包字符串"=w298:string)  [unwired: 10 in]
                            n275 = call "通信状态入队列.vi"("错误输入（无错误）"=w309, "发送报文"=w298, "枚举"=enum16{"打开连接", "发送数据", "读取数据", "数据处理", "关闭连接"}."发送数据") -> ()  [unwired: 8 in, 1 out]
                            n276 = Wait (ms)(milliseconds to wait=u32 1000 ("等待时间（毫秒）")) -> ()  [unwired: 1 out]
                          }
                        }
                      }
                    }
                    frame True {
                    }
                  }
                }
              }
            }
          }
          n277 = Not(x=w16) -> (.not. x?=w17:bool)
          n278 = global write "全局1.vi" "核查数据上传"(w17) -> ()
        }
        n279 = global read "断电保存全局.vi" "日志、参数发送"() -> (w14:bool)
        n280 = case shown="真" w14 {
          tunnel: ["环境参数" ("组合框") "操作日志" ("组合框")] -> w15
          frame False {
          }
          frame True {
          }
        }
      }
      frame "操作日志" {
        # "间隔时间上传"
        # "直接1分钟查询 一次,有数据就按数据上传,没数据就不上传,在数据发送那边有做处理"
        n281 = flat-sequence {
          frame #0 {
            # "时间"
            n282 = global write "全局 小时数据发送次数.vi" "小时数据发送次数"(0 ("小时数据发送次数")) -> ()
            n283 = call "日志信息主动发送(子VI).vi"() -> ()  [unwired: 12 in]
            n284 = global write "全局1.vi" "枚举"(enum16{"返回请求应答", "上传数据", "返回执行结果"}."上传数据" ("枚举")) -> ()
          }
          frame #1 {
            n285 = call "获取操作日志 (子VI).vi"("table输入"="操作日志") -> ()  [unwired: 11 in]
          }
          frame #2 {
            n286 = call "数据处理整合 (子VI).vi"("枚举"=enum16{"实时数据排序", "小时数据排序"}."实时数据排序") -> ("已排序的数组"=w324:string[])  [unwired: 10 in]
            n287 = Array Size(array=w324) -> (size(s)=w323:i32)
            n288 = global write "全局 数据数组大小.vi" "数据数组大小"(w323) -> ()
          }
          frame #3 {
            n289 = global read "全局 数据发送重叠.vi" "掉线指示灯"() -> (w326:bool)
            n290 = Not(x=w326) -> (.not. x?=w325:bool)
            n291 = case shown="真" w325 {
              frame False {
              }
              frame True {
                n292 = global read "全局 时间2.vi" "仪器日志索引"() -> (w330:T13)
                n293 = Cluster To Array(cluster=w330) -> (array=w329:string[])
                n294 = for {
                  tunnel: w329 -> [w331] mode=indexing
                  tunnel: [w332] -> w327 mode=indexing
                  i -> [w334]
                  # "行数大于零"
                  n295 = case shown="6" w334 {
                    tunnel: [w338 w339 w340 w341 w342 w343 w344] -> w333
                    frame 0, Default {
                      n296 = global read "全局 所有参数.vi" "氨氮"() -> (w338:string[][])
                    }
                    frame 1 {
                      n297 = global read "全局 所有参数.vi" "总磷"() -> (w339:string[][])
                    }
                    frame 2 {
                      n298 = global read "全局 所有参数.vi" "总氮"() -> (w340:string[][])
                    }
                    frame 3 {
                      n299 = global read "全局 所有参数.vi" "CODMn"() -> (w341:string[][])
                    }
                    frame 4 {
                      n300 = global read "全局 所有参数.vi" "CODCr"() -> (w342:string[][])
                    }
                    frame 5 {
                      n301 = global read "全局 所有参数.vi" "DO"() -> (w343:string[][])
                    }
                    frame 6 {
                      n302 = global read "全局 所有参数.vi" "氟化物"() -> (w344:string[][])
                    }
                  }
                  n303 = Array Size(array=w333) -> (size(s)=w336:i32[])
                  n304 = Index Array(array=w336) -> (element=w335:i32)  [unwired: 1 in]
                  n305 = Greater Than 0?(x=w335) -> (x > 0?=w337:bool)
                  n306 = case shown="真" w337 {
                    tunnel: w335 -> [_ _]
                    tunnel: w333 -> [_ w350]
                    tunnel: [w345 w346] -> w332
                    tunnel: w331 -> [w345 _]
                    frame False {
                    }
                    frame True {
                      # "最新时间戳加1分钟"
                      n307 = Array Size(array=w350) -> (size(s)=w352:i32[])
                      n308 = Index Array(array=w352) -> (element=w351:i32)  [unwired: 1 in]
                      n309 = Decrement(x=w351) -> (x-1=w349:i32)
                      n310 = Index Array(array=w350, index (row)=w349, index (col)=0 ("禁用的索引 (列)")) -> (element=w347:string)
                      n311 = call "日期时间字符串转换秒数加一.vi"("data[0]"=w347) -> ("日期/时间字符串"=w346:string)  [unwired: 10 in]
                    }
                  }
                }
                n312 = Array To Cluster(array=w327) -> (cluster=w328:T14)
                n313 = global write "全局 时间2.vi" "仪器日志索引"(w328) -> ()
              }
            }
          }
          frame #4 {
            # "判定是否存表"
            n314 = global read "全局 数据发送重叠.vi" "掉线指示灯"() -> (w353:bool)
            n315 = case shown="假" w353 {
              frame False {
                n316 = global read "全局 数据数组大小.vi" "数据数组大小"() -> (w354:i32)
                n317 = Greater Than 0?(x=w354) -> (x > 0?=w355:bool)
                n318 = case shown="真" w355 {
                  frame False {
                  }
                  frame True {
                    n319 = while {
                      stop <- w359 stop-if-true
                      n320 = Get Date/Time In Seconds() -> (seconds since 1Jan1904=w369:timestamp)
                      n321 = Format Date/Time String(time format string (%c)="%Y%m%d%H%M%S%3u" ("时间格式字符串(%c)"), seconds (now)=w369) -> (date/time string=w368:string)  [unwired: 1 in]
                      n322 = Search and Replace String(input string=w368, search string="." ("搜索字符串")) -> (result string=w366:string)  [unwired: 6 in, 3 out]
                      n323 = global read "断电保存全局.vi" "MN"() -> (w365:string)
                      n324 = global read "断电保存全局.vi" "PW"() -> (w364:string)
                      n325 = call "数据编码.vi"("table输入"="操作日志" ("新元素/子数组"), "QN"=w366, "MN"=w365, "PW"=w364) -> ("错误常量"=w363:errorcluster, "通讯包字符串"=w356:string)  [unwired: 10 in]
                      n326 = global read "全局 小时数据发送次数.vi" "小时数据发送次数"() -> (w360:i32)
                      n327 = global read "全局 数据数组大小.vi" "数据数组大小"() -> (w361:i32)
                      n328 = call "通信状态入队列.vi"("错误输入（无错误）"=w363, "发送报文"=w356, "枚举"=enum16{"打开连接", "发送数据", "读取数据", "数据处理", "关闭连接"}."发送数据") -> ()  [unwired: 8 in, 1 out]
                      n329 = Decrement(x=w361) -> (x-1=w362:i32)
                      n330 = Greater Or Equal?(x=w360, y=w362) -> (x >= y?=w359:bool)
                      n331 = Wait (ms)(milliseconds to wait=u32 1000 ("等待时间（毫秒）")) -> ()  [unwired: 1 out]
                    }
                  }
                }
              }
              frame True {
              }
            }
          }
        }
        n332 = global read "断电保存全局.vi" "应用环境"() -> (w316:enum16{"STD", "GB212"})
        n333 = case shown="\"STD\", 默认" w316 {
          tunnel: ["3092日志信息" ("组合框") "系统状态" ("组合框")] -> w315
          frame "STD", Default {
          }
          frame "GB212" {
          }
        }
      }
      frame "3092日志信息" {
        # "间隔时间上传"
        # "直接1分钟查询 一次,有数据就按数据上传,没数据就不上传,在数据发送那边有做处理"
        n334 = flat-sequence {
          tunnel: [w376] -> w372
          tunnel: w372 -> [w380]
          frame #0 {
            n335 = global write "全局 小时数据发送次数.vi" "小时数据发送次数"(0 ("小时数据发送次数")) -> ()
            n336 = global write "全局1.vi" "枚举"(enum16{"返回请求应答", "上传数据", "返回执行结果"}."上传数据" ("枚举")) -> ()
          }
          frame #1 {
            n337 = call "数据表比对.vi"("table输入"="3092日志信息") -> ("待发送数据"=w376:string[][])  [unwired: 7 in, 3 out]
            n338 = global write "全局 所有参数.vi" "CODMn"(w376) -> ()
          }
          frame #2 {
            n339 = Array Size(array=w380) -> (size(s)=w379:i32[])
            n340 = Index Array(array=w379) -> (element=w378:i32)  [unwired: 1 in]
            n341 = global write "全局 数据数组大小.vi" "数据数组大小"(w378) -> ()
          }
          frame #3 {
            n342 = global read "全局 数据发送重叠.vi" "掉线指示灯"() -> (w382:bool)
            n343 = Not(x=w382) -> (.not. x?=w381:bool)
            n344 = case shown="真" w381 {
              frame False {
              }
              frame True {
                # "行数大于零"
                n345 = global read "全局 时间2.vi" "3092日志索引起始时间"() -> (w384:string)
                n346 = global read "全局 所有参数.vi" "CODMn"() -> (w385:string[][])
                n347 = Array Size(array=w385) -> (size(s)=w387:i32[])
                n348 = Index Array(array=w387) -> (element=w386:i32)  [unwired: 1 in]
                n349 = Greater Than 0?(x=w386) -> (x > 0?=w388:bool)
                n350 = case shown="真" w388 {
                  tunnel: w386 -> [_ _]
                  tunnel: w385 -> [_ w394]
                  tunnel: [w389 w390] -> w383
                  tunnel: w384 -> [w389 _]
                  frame False {
                  }
                  frame True {
                    # "最新时间戳加1分钟"
                    n351 = Array Size(array=w394) -> (size(s)=w396:i32[])
                    n352 = Index Array(array=w396) -> (element=w395:i32)  [unwired: 1 in]
                    n353 = Decrement(x=w395) -> (x-1=w393:i32)
                    n354 = Index Array(array=w394, index (row)=w393, index (col)=0 ("禁用的索引 (列)")) -> (element=w391:string)
                    n355 = call "日期时间字符串转换秒数加一.vi"("data[0]"=w391) -> ("日期/时间字符串"=w390:string)  [unwired: 10 in]
                  }
                }
                n356 = global write "全局 时间2.vi" "3092日志索引起始时间"(w383) -> ()
              }
            }
          }
          frame #4 {
            # "判定是否存表"
            n357 = global read "全局 数据发送重叠.vi" "掉线指示灯"() -> (w397:bool)
            n358 = case shown="假" w397 {
              frame False {
                n359 = global read "全局 数据数组大小.vi" "数据数组大小"() -> (w398:i32)
                n360 = Greater Than 0?(x=w398) -> (x > 0?=w399:bool)
                n361 = case shown="真" w399 {
                  frame False {
                  }
                  frame True {
                    n362 = while {
                      stop <- w403 stop-if-true
                      n363 = global read "全局 数据数组大小.vi" "数据数组大小"() -> (w405:i32)
                      n364 = Wait (ms)(milliseconds to wait=u32 1000 ("等待时间（毫秒）")) -> ()  [unwired: 1 out]
                      n365 = global read "全局 小时数据发送次数.vi" "小时数据发送次数"() -> (w404:i32)
                      n366 = Decrement(x=w405) -> (x-1=w406:i32)
                      n367 = Greater Or Equal?(x=w404, y=w406) -> (x >= y?=w403:bool)
                      n368 = Get Date/Time In Seconds() -> (seconds since 1Jan1904=w413:timestamp)
                      n369 = Format Date/Time String(time format string (%c)="%Y%m%d%H%M%S%3u" ("时间格式字符串(%c)"), seconds (now)=w413) -> (date/time string=w412:string)  [unwired: 1 in]
                      n370 = Search and Replace String(input string=w412, search string="." ("搜索字符串")) -> (result string=w410:string)  [unwired: 6 in, 3 out]
                      n371 = global read "断电保存全局.vi" "MN"() -> (w409:string)
                      n372 = global read "断电保存全局.vi" "PW"() -> (w408:string)
                      n373 = call "数据编码.vi"("table输入"="3092日志信息" ("新元素/子数组"), "QN"=w410, "MN"=w409, "PW"=w408) -> ("错误常量"=w407:errorcluster, "通讯包字符串"=w400:string)  [unwired: 10 in]
                      n374 = call "通信状态入队列.vi"("错误输入（无错误）"=w407, "发送报文"=w400, "枚举"=enum16{"打开连接", "发送数据", "读取数据", "数据处理", "关闭连接"}."发送数据") -> ()  [unwired: 8 in, 1 out]
                    }
                  }
                }
              }
              frame True {
              }
            }
          }
        }
      }
      frame "系统状态" {
        # "直接1分钟查询 一次,有变化就按上传,没变化就不上传"
        n375 = flat-sequence {
          frame #0 {
            # "时间"
            n376 = global write "全局 小时数据发送次数.vi" "小时数据发送次数"(0 ("小时数据发送次数")) -> ()
            n377 = global write "全局 数据数组大小.vi" "数据数组大小"(1 ("数据数组大小")) -> ()
            n378 = global write "全局1.vi" "枚举"(enum16{"返回请求应答", "上传数据", "返回执行结果"}."上传数据" ("枚举")) -> ()
          }
          frame #1 {
            # "判定是否存表"
            n379 = global read "全局 数据发送重叠.vi" "掉线指示灯"() -> (w424:bool)
            n380 = case shown="假" w424 {
              frame False {
                n381 = global read "全局1.vi" "系统状态"() -> (w425:bool)
                n382 = case shown="真" w425 {
                  frame False {
                  }
                  frame True {
                    n383 = for {
                      N: 6 -> [_]
                      n384 = flat-sequence {
                        frame #0 {
                          n385 = Get Date/Time In Seconds() -> (seconds since 1Jan1904=w437:timestamp)
                          n386 = Format Date/Time String(time format string (%c)="%Y%m%d%H%M%S%3u" ("时间格式字符串(%c)"), seconds (now)=w437) -> (date/time string=w436:string)  [unwired: 1 in]
                          n387 = Search and Replace String(input string=w436, search string="." ("搜索字符串")) -> (result string=w434:string)  [unwired: 6 in, 3 out]
                          n388 = global read "断电保存全局.vi" "MN"() -> (w433:string)
                          n389 = global read "断电保存全局.vi" "PW"() -> (w432:string)
                          n390 = call "数据编码.vi"("table输入"="系统状态" ("新元素/子数组"), "QN"=w434, "MN"=w433, "PW"=w432) -> ("错误常量"=w431:errorcluster, "通讯包字符串"=w429:string)  [unwired: 10 in]
                          n391 = call "通信状态入队列.vi"("错误输入（无错误）"=w431, "发送报文"=w429, "枚举"=enum16{"打开连接", "发送数据", "读取数据", "数据处理", "关闭连接"}."发送数据") -> ()  [unwired: 8 in, 1 out]
                        }
                        frame #1 {
                          n392 = global read "全局 小时数据发送次数.vi" "小时数据发送次数"() -> (w441:i32)
                          n393 = Increment(x=w441) -> (x+1=w440:i32)
                          n394 = global write "全局 小时数据发送次数.vi" "小时数据发送次数"(w440) -> ()
                        }
                      }
                      n395 = Wait (ms)(milliseconds to wait=u32 1000 ("等待时间（毫秒）")) -> ()  [unwired: 1 out]
                    }
                    n396 = global write "全局1.vi" "系统状态"(FALSE ("系统状态")) -> ()
                  }
                }
              }
              frame True {
              }
            }
          }
        }
        n397 = global read "断电保存全局.vi" "应用环境"() -> (w416:enum16{"STD", "GB212"})
        n398 = case shown="\"STD\", 默认" w416 {
          tunnel: ["运行模式" ("组合框") "超标留样" ("组合框")] -> w417
          frame "STD", Default {
            n399 = global write "全局 数据发送重叠.vi" "数据接收超时指示灯"(FALSE ("数据接收超时指示灯")) -> ()
          }
          frame "GB212" {
          }
        }
      }
      frame "运行模式" {
        # "直接1分钟查询 一次,有变化就按上传,没变化就不上传"
        n400 = flat-sequence {
          frame #0 {
            # "时间"
            n401 = global write "全局 小时数据发送次数.vi" "小时数据发送次数"(0 ("小时数据发送次数")) -> ()
            n402 = global write "全局 数据数组大小.vi" "数据数组大小"(1 ("数据数组大小")) -> ()
            n403 = global write "全局1.vi" "枚举"(enum16{"返回请求应答", "上传数据", "返回执行结果"}."上传数据" ("枚举")) -> ()
          }
          frame #1 {
            # "判定是否存表"
            n404 = global read "全局 数据发送重叠.vi" "掉线指示灯"() -> (w446:bool)
            n405 = case shown="假" w446 {
              frame False {
                n406 = global read "全局1.vi" "运行模式"() -> (w447:bool)
                n407 = case shown="真" w447 {
                  frame False {
                  }
                  frame True {
                    n408 = global read "全局 小时数据发送次数.vi" "小时数据发送次数"() -> (w458:i32)
                    n409 = global write "全局1.vi" "运行模式"(FALSE ("系统状态")) -> ()
                    n410 = Get Date/Time In Seconds() -> (seconds since 1Jan1904=w461:timestamp)
                    n411 = Increment(x=w458) -> (x+1=w457:i32)
                    n412 = Format Date/Time String(time format string (%c)="%Y%m%d%H%M%S%3u" ("时间格式字符串(%c)"), seconds (now)=w461) -> (date/time string=w460:string)  [unwired: 1 in]
                    n413 = global write "全局 小时数据发送次数.vi" "小时数据发送次数"(w457) -> ()
                    n414 = Search and Replace String(input string=w460, search string="." ("搜索字符串")) -> (result string=w452:string)  [unwired: 6 in, 3 out]
                    n415 = global read "断电保存全局.vi" "MN"() -> (w456:string)
                    n416 = global read "断电保存全局.vi" "PW"() -> (w455:string)
                    n417 = call "数据编码.vi"("table输入"="运行模式" ("新元素/子数组"), "QN"=w452, "MN"=w456, "PW"=w455) -> ("错误常量"=w454:errorcluster, "通讯包字符串"=w448:string)  [unwired: 10 in]
                    n418 = call "通信状态入队列.vi"("错误输入（无错误）"=w454, "发送报文"=w448, "枚举"=enum16{"打开连接", "发送数据", "读取数据", "数据处理", "关闭连接"}."发送数据") -> ("错误输出"=w451:errorcluster)  [unwired: 8 in]
                    n419 = global read "断电保存全局.vi" "应用环境"() -> (w450:enum16{"STD", "GB212"})
                    n420 = case shown="\"STD\"" w450 {
                      tunnel: w452 -> [w467 _]
                      tunnel: w448 -> [w466 _]
                      tunnel: w451 -> [w465 _]
                      frame "STD" {
                        n421 = global read "断电保存全局.vi" "判断数据反馈"() -> (w464:enum16{"非严格判断", "严格判断", "不判断"})
                        n422 = case shown="\"严格判断\"" w464 {
                          tunnel: w466 -> [_ w472]
                          tunnel: w465 -> [_ w471]
                          tunnel: w467 -> [_ w470]
                          frame "不判断", Default {
                          }
                          frame "严格判断" {
                            n423 = global read "断电保存全局.vi" "数据发送通道"() -> (w469:enum16{"TCP", "VISA"})
                            n424 = call "数据补发判定有限循环.vi"("错误输入（无错误）"=w471, "数据输入"=w472, "QN"=w470, "数据发送通道"=w469) -> ("error out"=w468:errorcluster)  [unwired: 7 in]
                            n425 = case shown="无错误" w468 {
                              frame No Error {
                                n426 = global read "全局 数据发送重叠.vi" "数据接收超时指示灯"() -> (w473:bool)
                                n427 = case shown="真" w473 {
                                frame False {
                                }
                                frame True {
                                n428 = global write "全局1.vi" "测量周期"(TRUE ("测量周期")) -> ()
                                }
                                }
                              }
                              frame Error {
                              }
                            }
                          }
                        }
                      }
                      frame "GB212", Default {
                      }
                    }
                  }
                }
              }
              frame True {
              }
            }
          }
        }
      }
      frame "测量周期" {
        # "直接1分钟查询 一次,有变化就按上传,没变化就不上传"
        n429 = flat-sequence {
          frame #0 {
            # "时间"
            n430 = global write "全局 小时数据发送次数.vi" "小时数据发送次数"(0 ("小时数据发送次数")) -> ()
            n431 = global write "全局1.vi" "枚举"(enum16{"返回请求应答", "上传数据", "返回执行结果"}."上传数据" ("枚举")) -> ()
            n432 = global write "全局 数据数组大小.vi" "数据数组大小"(1 ("数据数组大小")) -> ()
          }
          frame #1 {
            # "判定是否存表"
            n433 = global read "全局 数据发送重叠.vi" "掉线指示灯"() -> (w479:bool)
            n434 = case shown="假" w479 {
              frame False {
                n435 = global read "全局1.vi" "测量周期"() -> (w480:bool)
                n436 = case shown="真" w480 {
                  frame False {
                  }
                  frame True {
                    n437 = global read "全局1.vi" "读取各参数测量周期的值"() -> (w488:u16[])
                    n438 = global write "全局1.vi" "测量周期"(FALSE ("系统状态")) -> ()
                    n439 = for {
                      tunnel: w488 -> [w533] mode=indexing
                      shift-right: [w531] -> w492
                      shift-left: u16[] [] ("读取各参数测量周期的值") -> [w534]
                      n440 = Not Equal To 0?(x=w533) -> (x != 0?=w532:bool)
                      n441 = case shown="真" w532 {
                        tunnel: w534 -> [w535 w538]
                        tunnel: w533 -> [_ w537]
                        tunnel: [w535 w536] -> w531
                        frame False {
                        }
                        frame True {
                          n442 = Insert Into Array(array=w538, new element=w537) -> (w536:u16[])  [unwired: 1 in]
                        }
                      }
                    }
                    n443 = global read "断电保存全局.vi" "应用环境"() -> (w485:enum16{"STD", "GB212"})
                    n444 = Array Max & Min(array=w492) -> (max value=w491:u16, min value=w490:u16)  [unwired: 2 out]
                    n445 = Not Equal?(x=w491, y=w490) -> (x != y?=w493:bool)
                    n446 = Equal?(x=w485, y=enum16{"STD", "GB212"}."STD") -> (x = y?=w487:bool)
                    n447 = And(x=w493, y=w487) -> (x .and. y?=w494:bool)
                    n448 = case shown="真" w494 {
                      tunnel: [w510 w522] -> w483
                      tunnel: [w509 w521] -> w482
                      tunnel: [w507 w519] -> w481
                      frame False {
                        n449 = Get Date/Time In Seconds() -> (seconds since 1Jan1904=w516:timestamp)
                        n450 = Format Date/Time String(time format string (%c)="%Y%m%d%H%M%S%3u" ("时间格式字符串(%c)"), seconds (now)=w516) -> (date/time string=w515:string)  [unwired: 1 in]
                        n451 = Search and Replace String(input string=w515, search string="." ("搜索字符串")) -> (result string=w509:string)  [unwired: 6 in, 3 out]
                        n452 = global read "断电保存全局.vi" "MN"() -> (w513:string)
                        n453 = global read "断电保存全局.vi" "PW"() -> (w512:string)
                        n454 = call "数据编码.vi"("table输入"="测量周期" ("新元素/子数组"), "QN"=w509, "MN"=w513, "PW"=w512) -> ("错误常量"=w511:errorcluster, "通讯包字符串"=w507:string)  [unwired: 10 in]
                        n455 = call "通信状态入队列.vi"("错误输入（无错误）"=w511, "发送报文"=w507, "枚举"=enum16{"打开连接", "发送数据", "读取数据", "数据处理", "关闭连接"}."发送数据") -> ("错误输出"=w510:errorcluster)  [unwired: 8 in]
                      }
                      frame True {
                        # "STD&参数测量周期不一样"
                        n456 = Get Date/Time In Seconds() -> (seconds since 1Jan1904=w528:timestamp)
                        n457 = Format Date/Time String(time format string (%c)="%Y%m%d%H%M%S%3u" ("时间格式字符串(%c)"), seconds (now)=w528) -> (date/time string=w527:string)  [unwired: 1 in]
                        n458 = Search and Replace String(input string=w527, search string="." ("搜索字符串")) -> (result string=w521:string)  [unwired: 6 in, 3 out]
                        n459 = global read "断电保存全局.vi" "MN"() -> (w525:string)
                        n460 = global read "断电保存全局.vi" "PW"() -> (w524:string)
                        n461 = call "数据编码.vi"("table输入"="各参数测量周期" ("新元素/子数组"), "QN"=w521, "MN"=w525, "PW"=w524) -> ("错误常量"=w523:errorcluster, "通讯包字符串"=w519:string)  [unwired: 10 in]
                        n462 = call "通信状态入队列.vi"("错误输入（无错误）"=w523, "发送报文"=w519, "枚举"=enum16{"打开连接", "发送数据", "读取数据", "数据处理", "关闭连接"}."发送数据") -> ("错误输出"=w522:errorcluster)  [unwired: 8 in]
                      }
                    }
                    n463 = global read "断电保存全局.vi" "应用环境"() -> (w484:enum16{"STD", "GB212"})
                    n464 = case shown="\"STD\"" w484 {
                      tunnel: w482 -> [w499 _]
                      tunnel: w481 -> [w498 _]
                      tunnel: w483 -> [w497 _]
                      frame "STD" {
                        n465 = global read "断电保存全局.vi" "判断数据反馈"() -> (w496:enum16{"非严格判断", "严格判断", "不判断"})
                        n466 = case shown="\"严格判断\"" w496 {
                          tunnel: w498 -> [_ w504]
                          tunnel: w497 -> [_ w503]
                          tunnel: w499 -> [_ w502]
                          frame "不判断", Default {
                          }
                          frame "严格判断" {
                            n467 = global read "断电保存全局.vi" "数据发送通道"() -> (w501:enum16{"TCP", "VISA"})
                            n468 = call "数据补发判定有限循环.vi"("错误输入（无错误）"=w503, "数据输入"=w504, "QN"=w502, "数据发送通道"=w501) -> ("error out"=w500:errorcluster)  [unwired: 7 in]
                            n469 = case shown="无错误" w500 {
                              frame No Error {
                                n470 = global read "全局 数据发送重叠.vi" "数据接收超时指示灯"() -> (w505:bool)
                                n471 = case shown="真" w505 {
                                frame False {
                                }
                                frame True {
                                n472 = global write "全局1.vi" "测量周期"(TRUE ("测量周期")) -> ()
                                }
                                }
                              }
                              frame Error {
                              }
                            }
                          }
                        }
                      }
                      frame "GB212", Default {
                      }
                    }
                  }
                }
              }
              frame True {
              }
            }
          }
        }
      }
      frame "超标留样" {
        # "直接1分钟查询 一次,有变化就按上传,没变化就不上传"
        n473 = flat-sequence {
          frame #0 {
            # "时间"
            n474 = global write "全局 小时数据发送次数.vi" "小时数据发送次数"(0 ("小时数据发送次数")) -> ()
            n475 = global write "全局 数据数组大小.vi" "数据数组大小"(1 ("数据数组大小")) -> ()
            n476 = global write "全局1.vi" "枚举"(enum16{"返回请求应答", "上传数据", "返回执行结果"}."上传数据" ("枚举")) -> ()
          }
          frame #1 {
            # "判定是否存表"
            n477 = global read "全局 数据发送重叠.vi" "掉线指示灯"() -> (w543:bool)
            n478 = case shown="假" w543 {
              frame False {
                n479 = global read "全局1.vi" "超标留样"() -> (w544:bool)
                n480 = case shown="真" w544 {
                  frame False {
                  }
                  frame True {
                    n481 = global read "全局 小时数据发送次数.vi" "小时数据发送次数"() -> (w552:i32)
                    n482 = global write "全局1.vi" "超标留样"(FALSE ("系统状态")) -> ()
                    n483 = Get Date/Time In Seconds() -> (seconds since 1Jan1904=w556:timestamp)
                    n484 = Increment(x=w552) -> (x+1=w551:i32)
                    n485 = Format Date/Time String(time format string (%c)="%Y%m%d%H%M%S%3u" ("时间格式字符串(%c)"), seconds (now)=w556) -> (date/time string=w555:string)  [unwired: 1 in]
                    n486 = global write "全局 小时数据发送次数.vi" "小时数据发送次数"(w551) -> ()
                    n487 = Search and Replace String(input string=w555, search string="." ("搜索字符串")) -> (result string=w553:string)  [unwired: 6 in, 3 out]
                    n488 = global read "断电保存全局.vi" "MN"() -> (w549:string)
                    n489 = global read "断电保存全局.vi" "PW"() -> (w548:string)
                    n490 = call "数据编码.vi"("table输入"="超标留样" ("新元素/子数组"), "QN"=w553, "MN"=w549, "PW"=w548) -> ("错误常量"=w550:errorcluster, "通讯包字符串"=w545:string)  [unwired: 10 in]
                    n491 = call "通信状态入队列.vi"("错误输入（无错误）"=w550, "发送报文"=w545, "枚举"=enum16{"打开连接", "发送数据", "读取数据", "数据处理", "关闭连接"}."发送数据") -> ()  [unwired: 8 in, 1 out]
                  }
                }
              }
              frame True {
              }
            }
          }
        }
      }
      frame "报警信息" {
        # "间隔时间上传"
        # "直接1分钟查询 一次,有数据就按数据上传,没数据为空的不传,在数据发送那边有做处理"
        n492 = flat-sequence {
          frame #0 {
            # "分钟时间间隔"
            n493 = call "日志信息主动发送(子VI).vi"() -> ()  [unwired: 12 in]
            n494 = global write "全局 小时数据发送次数.vi" "小时数据发送次数"(0 ("小时数据发送次数")) -> ()
            n495 = global write "全局1.vi" "枚举"(enum16{"返回请求应答", "上传数据", "返回执行结果"}."上传数据" ("枚举")) -> ()
          }
          frame #1 {
            n496 = call "获取报警信息 (子VI).vi"() -> ()  [unwired: 12 in]
          }
          frame #2 {
            n497 = call "数据处理整合 (子VI).vi"("枚举"=enum16{"实时数据排序", "小时数据排序"}."实时数据排序") -> ("已排序的数组"=w570:string[])  [unwired: 10 in]
            n498 = Array Size(array=w570) -> (size(s)=w569:i32)
            n499 = global write "全局 数据数组大小.vi" "数据数组大小"(w569) -> ()
          }
          frame #3 {
            n500 = global read "全局 数据发送重叠.vi" "掉线指示灯"() -> (w572:bool)
            n501 = Not(x=w572) -> (.not. x?=w571:bool)
            n502 = case shown="真" w571 {
              frame False {
              }
              frame True {
                n503 = global read "全局 时间2.vi" "报警信息索引"() -> (w576:T15)
                n504 = Cluster To Array(cluster=w576) -> (array=w575:string[])
                n505 = for {
                  tunnel: [w578] -> w573 mode=indexing
                  tunnel: w575 -> [w577] mode=indexing
                  i -> [w580]
                  # "行数大于零"
                  n506 = case shown="12" w580 {
                    tunnel: [w584 w585 w586 w587 w588 w589 w590 w591 w592 w593 w594 w595 w596] -> w579
                    frame 0, Default {
                      n507 = global read "全局 所有参数.vi" "氨氮"() -> (w584:string[][])
                    }
                    frame 1 {
                      n508 = global read "全局 所有参数.vi" "总磷"() -> (w585:string[][])
                    }
                    frame 2 {
                      n509 = global read "全局 所有参数.vi" "总氮"() -> (w586:string[][])
                    }
                    frame 3 {
                      n510 = global read "全局 所有参数.vi" "CODMn"() -> (w587:string[][])
                    }
                    frame 4 {
                      n511 = global read "全局 所有参数.vi" "CODCr"() -> (w588:string[][])
                    }
                    frame 5 {
                      n512 = global read "全局 所有参数.vi" "DO"() -> (w589:string[][])
                    }
                    frame 6 {
                      n513 = global read "全局 所有参数.vi" "PH"() -> (w590:string[][])
                    }
                    frame 7 {
                      n514 = global read "全局 所有参数.vi" "电导率"() -> (w591:string[][])
                    }
                    frame 8 {
                      n515 = global read "全局 所有参数.vi" "水温"() -> (w592:string[][])
                    }
                    frame 9 {
                      n516 = global read "全局 所有参数.vi" "浊度"() -> (w593:string[][])
                    }
                    frame 10 {
                      n517 = global read "全局 所有参数.vi" "叶绿素"() -> (w594:string[][])
                    }
                    frame 11 {
                      n518 = global read "全局 所有参数.vi" "藻密度"() -> (w595:string[][])
                    }
                    frame 12 {
                      n519 = global read "全局 所有参数.vi" "氟化物"() -> (w596:string[][])
                    }
                  }
                  n520 = Array Size(array=w579) -> (size(s)=w582:i32[])
                  n521 = Index Array(array=w582) -> (element=w581:i32)  [unwired: 1 in]
                  n522 = Greater Than 0?(x=w581) -> (x > 0?=w583:bool)
                  n523 = case shown="真" w583 {
                    tunnel: w581 -> [_ _]
                    tunnel: w579 -> [_ w601]
                    tunnel: [w597 w598] -> w578
                    tunnel: w577 -> [w597 _]
                    frame False {
                    }
                    frame True {
                      # "最新时间戳加1分钟"
                      n524 = Array Size(array=w601) -> (size(s)=w603:i32[])
                      n525 = Index Array(array=w603) -> (element=w602:i32)  [unwired: 1 in]
                      n526 = Decrement(x=w602) -> (x-1=w600:i32)
                      n527 = Index Array(array=w601, index (row)=w600, index (col)=0 ("禁用的索引 (列)")) -> (element=w604:string)
                      n528 = call "日期时间字符串转换分钟数加一.vi"("data[0]"=w604) -> ("日期/时间字符串"=w598:string)  [unwired: 10 in]
                    }
                  }
                }
                n529 = Array To Cluster(array=w573) -> (cluster=w574:T16)
                n530 = global write "全局 时间2.vi" "报警信息索引"(w574) -> ()
              }
            }
          }
          frame #4 {
            # "判定是否存表"
            n531 = global read "全局 数据发送重叠.vi" "掉线指示灯"() -> (w605:bool)
            n532 = case shown="假" w605 {
              frame False {
                # "判定数据不为空才发"
                n533 = global read "全局 数据数组大小.vi" "数据数组大小"() -> (w606:i32)
                n534 = Greater Than 0?(x=w606) -> (x > 0?=w607:bool)
                n535 = case shown="真" w607 {
                  frame False {
                    n536 = global write "全局1.vi" "核查数据上传"(FALSE ("数据上传")) -> ()
                  }
                  frame True {
                    n537 = while {
                      stop <- w612 stop-if-true
                      n538 = Wait (ms)(milliseconds to wait=u32 1000 ("等待时间（毫秒）")) -> ()  [unwired: 1 out]
                      n539 = Get Date/Time In Seconds() -> (seconds since 1Jan1904=w622:timestamp)
                      n540 = Format Date/Time String(time format string (%c)="%Y%m%d%H%M%S%3u" ("时间格式字符串(%c)"), seconds (now)=w622) -> (date/time string=w621:string)  [unwired: 1 in]
                      n541 = global read "全局 数据数组大小.vi" "数据数组大小"() -> (w614:i32)
                      n542 = Search and Replace String(input string=w621, search string="." ("搜索字符串")) -> (result string=w619:string)  [unwired: 6 in, 3 out]
                      n543 = global read "断电保存全局.vi" "PW"() -> (w617:string)
                      n544 = global read "断电保存全局.vi" "MN"() -> (w618:string)
                      n545 = global read "全局 小时数据发送次数.vi" "小时数据发送次数"() -> (w615:i32)
                      n546 = call "数据编码.vi"("table输入"="报警信息" ("新元素/子数组"), "QN"=w619, "MN"=w618, "PW"=w617) -> ("错误常量"=w616:errorcluster, "通讯包字符串"=w609:string)  [unwired: 10 in]
                      n547 = Decrement(x=w614) -> (x-1=w613:i32)
                      n548 = Greater Or Equal?(x=w615, y=w613) -> (x >= y?=w612:bool)
                      n549 = call "通信状态入队列.vi"("错误输入（无错误）"=w616, "发送报文"=w609, "枚举"=enum16{"打开连接", "发送数据", "读取数据", "数据处理", "关闭连接"}."发送数据") -> ()  [unwired: 8 in, 1 out]
                    }
                  }
                }
              }
              frame True {
              }
            }
          }
        }
        n550 = global read "断电保存全局.vi" "应用环境"() -> (w560:enum16{"STD", "GB212"})
        n551 = case shown="\"GB212\"" w560 {
          tunnel: ["3093报警信息" ("组合框") w563] -> w559
          frame "STD", Default {
          }
          frame "GB212" {
            n552 = global read "断电保存全局.vi" "仪器参数发送"() -> (w562:bool)
            n553 = case shown="真" w562 {
              tunnel: ["环境参数" ("组合框") "仪器参数" ("组合框")] -> w563
              frame False {
              }
              frame True {
              }
            }
          }
        }
      }
      frame "3093报警信息" {
        # "间隔时间上传"
        # "直接1分钟查询 一次,有数据就按数据上传,没数据为空的不传,在数据发送那边有做处理"
        n554 = flat-sequence {
          tunnel: [w632] -> w627
          tunnel: w627 -> [w636]
          frame #0 {
            n555 = global write "全局 小时数据发送次数.vi" "小时数据发送次数"(0 ("小时数据发送次数")) -> ()
            n556 = global write "全局1.vi" "枚举"(enum16{"返回请求应答", "上传数据", "返回执行结果"}."上传数据" ("枚举")) -> ()
          }
          frame #1 {
            n557 = call "数据表比对.vi"("table输入"="3093报警信息") -> ("待发送数据"=w632:string[][])  [unwired: 7 in, 3 out]
            n558 = global write "全局 所有参数.vi" "CODMn"(w632) -> ()
          }
          frame #2 {
            n559 = Array Size(array=w636) -> (size(s)=w635:i32[])
            n560 = Index Array(array=w635) -> (element=w634:i32)  [unwired: 1 in]
            n561 = global write "全局 数据数组大小.vi" "数据数组大小"(w634) -> ()
          }
          frame #3 {
            n562 = global read "全局 数据发送重叠.vi" "掉线指示灯"() -> (w638:bool)
            n563 = Not(x=w638) -> (.not. x?=w637:bool)
            n564 = case shown="真" w637 {
              frame False {
              }
              frame True {
                # "行数大于零"
                n565 = global read "全局 时间2.vi" "3093报警索引起始时间"() -> (w640:string)
                n566 = global read "全局 所有参数.vi" "CODMn"() -> (w641:string[][])
                n567 = Array Size(array=w641) -> (size(s)=w643:i32[])
                n568 = Index Array(array=w643) -> (element=w642:i32)  [unwired: 1 in]
                n569 = Greater Than 0?(x=w642) -> (x > 0?=w644:bool)
                n570 = case shown="真" w644 {
                  tunnel: w642 -> [_ _]
                  tunnel: w641 -> [_ w650]
                  tunnel: [w645 w646] -> w639
                  tunnel: w640 -> [w645 _]
                  frame False {
                  }
                  frame True {
                    # "最新时间戳加1分钟"
                    n571 = Array Size(array=w650) -> (size(s)=w652:i32[])
                    n572 = Index Array(array=w652) -> (element=w651:i32)  [unwired: 1 in]
                    n573 = Decrement(x=w651) -> (x-1=w649:i32)
                    n574 = Index Array(array=w650, index (row)=w649, index (col)=0 ("禁用的索引 (列)")) -> (element=w647:string)
                    n575 = call "日期时间字符串转换秒数加一.vi"("data[0]"=w647) -> ("日期/时间字符串"=w646:string)  [unwired: 10 in]
                  }
                }
                n576 = global write "全局 时间2.vi" "3093报警索引起始时间"(w639) -> ()
              }
            }
          }
          frame #4 {
            # "判定是否存表"
            n577 = global read "全局 数据发送重叠.vi" "掉线指示灯"() -> (w653:bool)
            n578 = case shown="假" w653 {
              frame False {
                n579 = global read "全局 数据数组大小.vi" "数据数组大小"() -> (w654:i32)
                n580 = Greater Than 0?(x=w654) -> (x > 0?=w655:bool)
                n581 = case shown="真" w655 {
                  frame False {
                  }
                  frame True {
                    n582 = while {
                      stop <- w659 stop-if-true
                      n583 = global read "全局 数据数组大小.vi" "数据数组大小"() -> (w661:i32)
                      n584 = Wait (ms)(milliseconds to wait=u32 1000 ("等待时间（毫秒）")) -> ()  [unwired: 1 out]
                      n585 = global read "全局 小时数据发送次数.vi" "小时数据发送次数"() -> (w660:i32)
                      n586 = Decrement(x=w661) -> (x-1=w662:i32)
                      n587 = Greater Or Equal?(x=w660, y=w662) -> (x >= y?=w659:bool)
                      n588 = Get Date/Time In Seconds() -> (seconds since 1Jan1904=w669:timestamp)
                      n589 = Format Date/Time String(time format string (%c)="%Y%m%d%H%M%S%3u" ("时间格式字符串(%c)"), seconds (now)=w669) -> (date/time string=w668:string)  [unwired: 1 in]
                      n590 = Search and Replace String(input string=w668, search string="." ("搜索字符串")) -> (result string=w666:string)  [unwired: 6 in, 3 out]
                      n591 = global read "断电保存全局.vi" "MN"() -> (w665:string)
                      n592 = global read "断电保存全局.vi" "PW"() -> (w664:string)
                      n593 = call "数据编码.vi"("table输入"="3093报警信息" ("新元素/子数组"), "QN"=w666, "MN"=w665, "PW"=w664) -> ("错误常量"=w663:errorcluster, "通讯包字符串"=w656:string)  [unwired: 10 in]
                      n594 = call "通信状态入队列.vi"("错误输入（无错误）"=w663, "发送报文"=w656, "枚举"=enum16{"打开连接", "发送数据", "读取数据", "数据处理", "关闭连接"}."发送数据") -> ()  [unwired: 8 in, 1 out]
                    }
                  }
                }
              }
              frame True {
              }
            }
          }
        }
        n595 = global read "断电保存全局.vi" "仪器参数发送"() -> (w626:bool)
        n596 = case shown="真" w626 {
          tunnel: ["环境参数" ("组合框") "仪器参数" ("组合框")] -> w625
          frame False {
          }
          frame True {
          }
        }
      }
      frame "仪器参数" {
        n597 = flat-sequence {
          frame #0 {
            n598 = global write "全局 小时数据发送次数.vi" "小时数据发送次数"(0 ("小时数据发送次数")) -> ()
            n599 = global write "全局1.vi" "枚举"(enum16{"返回请求应答", "上传数据", "返回执行结果"}."上传数据" ("枚举")) -> ()
          }
          frame #1 {
            n600 = call "获取操作日志 (子VI).vi"("table输入"="仪器参数") -> ()  [unwired: 11 in]
          }
          frame #2 {
            n601 = global read "全局 数据发送重叠.vi" "掉线指示灯"() -> (w677:bool)
            n602 = Not(x=w677) -> (.not. x?=w676:bool)
            n603 = case shown="真" w676 {
              frame False {
              }
              frame True {
                n604 = global read "全局 时间2.vi" "仪器参数索引"() -> (w681:T17)
                n605 = Cluster To Array(cluster=w681) -> (array=w680:string[])
                n606 = for {
                  tunnel: [w685] -> w678 mode=indexing
                  tunnel: w680 -> [w684] mode=indexing
                  i -> [w683]
                  # "行数大于零"
                  n607 = case shown="0, 默认" w683 {
                    tunnel: [w689 w690 w691 w692 w693 w694 w695 w696 w697 w698 w699 w700 w701 w702] -> w682
                    frame 0, Default {
                      n608 = global read "全局 所有参数.vi" "氨氮"() -> (w689:string[][])
                    }
                    frame 1 {
                      n609 = global read "全局 所有参数.vi" "总磷"() -> (w690:string[][])
                    }
                    frame 2 {
                      n610 = global read "全局 所有参数.vi" "总氮"() -> (w691:string[][])
                    }
                    frame 3 {
                      n611 = global read "全局 所有参数.vi" "CODMn"() -> (w692:string[][])
                    }
                    frame 4 {
                      n612 = global read "全局 所有参数.vi" "CODCr"() -> (w693:string[][])
                    }
                    frame 5 {
                      n613 = global read "全局 所有参数.vi" "DO"() -> (w694:string[][])
                    }
                    frame 6 {
                      n614 = global read "全局 所有参数.vi" "PH"() -> (w695:string[][])
                    }
                    frame 7 {
                      n615 = global read "全局 所有参数.vi" "电导率"() -> (w696:string[][])
                    }
                    frame 8 {
                      n616 = global read "全局 所有参数.vi" "水温"() -> (w697:string[][])
                    }
                    frame 9 {
                      n617 = global read "全局 所有参数.vi" "浊度"() -> (w698:string[][])
                    }
                    frame 10 {
                      n618 = global read "全局 所有参数.vi" "叶绿素"() -> (w699:string[][])
                    }
                    frame 11 {
                      n619 = global read "全局 所有参数.vi" "藻密度"() -> (w700:string[][])
                    }
                    frame 12 {
                      n620 = global read "全局 所有参数.vi" "ORP"() -> (w701:string[][])
                    }
                    frame 13 {
                      n621 = global read "全局 所有参数.vi" "氟化物"() -> (w702:string[][])
                    }
                  }
                  n622 = Array Size(array=w682) -> (size(s)=w687:i32[])
                  n623 = Index Array(array=w687) -> (element=w686:i32)  [unwired: 1 in]
                  n624 = Greater Than 0?(x=w686) -> (x > 0?=w688:bool)
                  n625 = case shown="真" w688 {
                    tunnel: w686 -> [_ _]
                    tunnel: w682 -> [_ w708]
                    tunnel: [w703 w705] -> w685
                    tunnel: w684 -> [w703 _]
                    frame False {
                    }
                    frame True {
                      # "最新时间戳加1秒"
                      n626 = Array Size(array=w708) -> (size(s)=w710:i32[])
                      n627 = Index Array(array=w710) -> (element=w709:i32)  [unwired: 1 in]
                      n628 = Decrement(x=w709) -> (x-1=w707:i32)
                      n629 = Index Array(array=w708, index (row)=w707, index (col)=0 ("禁用的索引 (列)")) -> (element=w711:string)
                      n630 = call "日期时间字符串转换分钟数加一.vi"("枚举"=enum16{"分钟数加一", "秒数加一", "小时数加一"}."秒数加一", "data[0]"=w711) -> ("日期/时间字符串"=w705:string)  [unwired: 9 in]
                    }
                  }
                }
                n631 = Array To Cluster(array=w678) -> (cluster=w679:T18)
                n632 = global write "全局 时间2.vi" "仪器参数索引"(w679) -> ()
              }
            }
          }
          frame #3 {
            n633 = global read "全局 数据发送重叠.vi" "掉线指示灯"() -> (w713:bool)
            n634 = Not(x=w713) -> (.not. x?=w712:bool)
            n635 = case shown="真" w712 {
              frame False {
              }
              frame True {
                n636 = call "3020仪器参数发送.vi"() -> ()  [unwired: 12 in]
              }
            }
          }
        }
      }
      frame "环境参数", Default {
        n637 = call "核查数据断电保存 (子VI).vi"() -> ()  [unwired: 12 in]
      }
    }
  }
  "错误输出" <- w2
